vi "MBDoE3ParamAmb.vi"() -> ()   [LabVIEW 2015]
uses:
  <vilib>/Platform/TimedLoop/XDataNode/timing_clust.ctl
  <vilib>/Platform/TimedLoop/XDataNode/nitl_modes.ctl
  <vilib>/Platform/TimedLoop/XDataNode/wakeup.ctl
  <vilib>/DAQmx/read.llb/DAQmx Read (Analog DBL 1Chan 1Samp).vi
  <vilib>/DAQmx/read.llb/DAQmx Read (Analog 1D DBL NChan 1Samp).vi
  <vilib>/DAQmx/create/channels.llb/DAQmx Create Channel (AI-Voltage-Basic).vi
  <vilib>/Enthought/Python Integration Toolkit/api/Unpack Double.vi
  <vilib>/DAQmx/miscellaneous.llb/DAQmx Fill In Error Info.vi
  <vilib>/Platform/TimedLoop/XDataNode/XDataNode.xnode
  Program Files/neMESYS_SDK/neMESYS LabVIEW Kit/neMESYS LabVIEW Integration Kit.lvlib
  <vilib>/Platform/TimedLoop/XDataNode/XDNodeRunTimeDep.lvlib
  Conor/Temp CN7500/Omega CN7500/Omega CN7500.lvlib
  <vilib>/Enthought/Python Integration Toolkit/Python Integration Toolkit.lvlib
panel:
  in  "MBDoE Criteria A/D/E":string
  out "Record filename, RecordAmbInitisileFactorial1MD":string
  out "HPLC file name, MBDoE2peakin1":string
  out "Exp 9":bool
  out "Temp 9":dbl
  out "Flow 9":dbl
  out "Conc 9":dbl
  out "t1 - 8":dbl
  out "X2 ref A 8":dbl
  out "X2 B 8":dbl
  out "X ref B 8":dbl
  out "C BAcid 8":dbl
  out "C EB 8":dbl
  out "Exp 8":bool
  out "Temp 8":dbl
  out "Flow 8":dbl
  out "Conc 8":dbl
  out "t1 - 7":dbl
  out "X2 ref A 7":dbl
  out "X2 B 7":dbl
  out "X ref B 7":dbl
  out "C BAcid 7":dbl
  out "C EB 7":dbl
  out "Exp 7":bool
  out "Temp 7":dbl
  out "Flow 7":dbl
  out "Conc 7":dbl
  out "t1 - 6":dbl
  out "X2 ref A 6":dbl
  out "X2 B 6":dbl
  out "X ref B 6":dbl
  out "C BAcid 6":dbl
  out "C EB 6":dbl
  out "Exp 6":bool
  out "Temp 6":dbl
  out "Flow 6":dbl
  out "Conc 6":dbl
  out "t1 - 5":dbl
  out "X2 ref A 5":dbl
  out "X2 B 5":dbl
  out "X ref B 5":dbl
  out "C BAcid 5":dbl
  out "C EB 5":dbl
  out "Exp 5":bool
  out "Temp 5":dbl
  out "Flow 5":dbl
  out "Conc 5":dbl
  out "t1 - 4":dbl
  out "X2 ref A 4":dbl
  out "X2 B 4":dbl
  out "X ref B 4":dbl
  out "C BAcid 4":dbl
  out "C EB 4":dbl
  out "Exp 4":bool
  out "Temp 4":dbl
  out "Flow 4":dbl
  out "Conc 4":dbl
  out "t1 - 3":dbl
  out "X2 ref A 3":dbl
  out "X2 B 3":dbl
  out "X ref B 3":dbl
  out "C BAcid 3":dbl
  out "C EB 3":dbl
  out "Exp 3":bool
  out "Temp 3":dbl
  out "Flow 3":dbl
  out "Conc 3":dbl
  out "t1 2":dbl
  out "X2 ref A 2":dbl
  out "X2 B 2":dbl
  out "X ref B 2":dbl
  out "C BAcid 2":dbl
  out "C EB 2":dbl
  in  "Cat Mass (0.096 g)":dbl
  in  "Cat Diameter (825 um)":dbl
  out "t1 - 1":dbl
  out "X2 ref A 1":dbl
  out "X2 B 1":dbl
  out "X ref B 1":dbl
  out "Exp 1":bool
  out "C EB 1":dbl
  out "C BAcid 1":dbl
  out "Liquid Inlet Pressure (bar g)":dbl
  in  "Liquid P sensor Terminal Configuration":i32(ring)=-1 items=["default"=-1, "RSE"=10083, "NRSE"=10078, "Differential"=10106, "Pseudodifferential"=12529]
  in  "Liquid P sensor Physical Channel":tag="Dev1/ai0"
  out "Exp 2":bool
  out "Exp 0":bool
  out "Conc 1":dbl
  out "Flow 1":dbl
  out "Temp 1":dbl
  out "Conc 2":dbl
  out "Flow 2":dbl
  out "Temp 2":dbl
  out "t1":dbl
  out "t2":dbl
  out "t3":dbl
  out "tref":dbl
  out "Desired Conc Not Possible":bool
  in  "Safety or Emergency Syringe Control":bool
  out "Feed Concentration (M)":dbl
  out "Total Flowrate (uL/min)":dbl
  out "Gas Back Pressure (barg)":dbl
  in  "Shut down in empty?\nLeft off, right on":bool
  in  "Clear":bool
  out "Safety Shut Down Pressure (barg)":dbl
  out "Calculated Pressure":dbl[](graph)
  out "Safety Shut Down Temp":dbl
  out "Actual Temp (oC)":dbl
  out "Temperature":dynamicdata(graph)
  out "Temp Set Point (oC)":dbl
  in  "Temp 0":dbl
  in  "Update Temperature Set Point":bool
  in  "Automated Experiments or Direct Control":bool
  in  "Set Point (oC)":dbl
  out "loop ind":dbl
  in  "Stop everything":bool
  in  "Skip Exp":bool
  in  "Minutes between Exp":dbl min=0.0 step=0.05
  in  "Refill 4":bool
  in  "Refill 3":bool
  in  "Refill 2":bool
  in  "Refill 1":bool
  in  "Empty 4":bool
  in  "Empty 3":bool
  in  "Empty 2":bool
  in  "Empty 1":bool
  in  "Calibrate 4":bool
  in  "Calibrate 3":bool
  in  "Calibrate 2":bool
  in  "Calibrate 1":bool
  in  "Stop Dose 4":bool
  in  "Stop Dose 3":bool
  in  "Stop Dose 2":bool
  in  "Stop Dose 1":bool
  in  "Flow 0":dbl
  in  "Conc 0":dbl
  in  "Generate Flow":bool
  in  "Set Flowrate 1":dbl
  in  "Set Flowrate 2":dbl
  in  "Set Flowrate 3":dbl
  in  "Set Flowrate 4":dbl
  in  "High Conc":dbl min=0.0 max=2.0
  in  "Low Conc":dbl min=0.0 max=2.0
  out "Syringe Level 4":dbl(slide) scale=0.0..5500.0
  out "Syringe Level 3":dbl(slide) scale=0.0..5500.0
  out "Syringe Level 2":dbl(slide) scale=0.0..5500.0
  out "Syringe Level 1":dbl(slide) scale=0.0..5500.0
  out "Flowrate 4 High":dbl
  out "Flowrate 3 High":dbl
  out "Flowrate 2 Low":dbl
  out "Flowrate 1 Low":dbl
  # "Pre Planned Experiments"
  # "Conducted Experiments Set Points"
  # "Safety (start and end)"
  # "Current Conditions"
  # "(uL/min)"
  # "Coerced to nearest possible"
  # "Experimental Info"
  # "This code only does Automated \nDirect control just sets all variables to 0"
  # "Direct Control"
  # "Unit of Gas Flow NmL/min"
  # "Emergency Syringe Control Below"
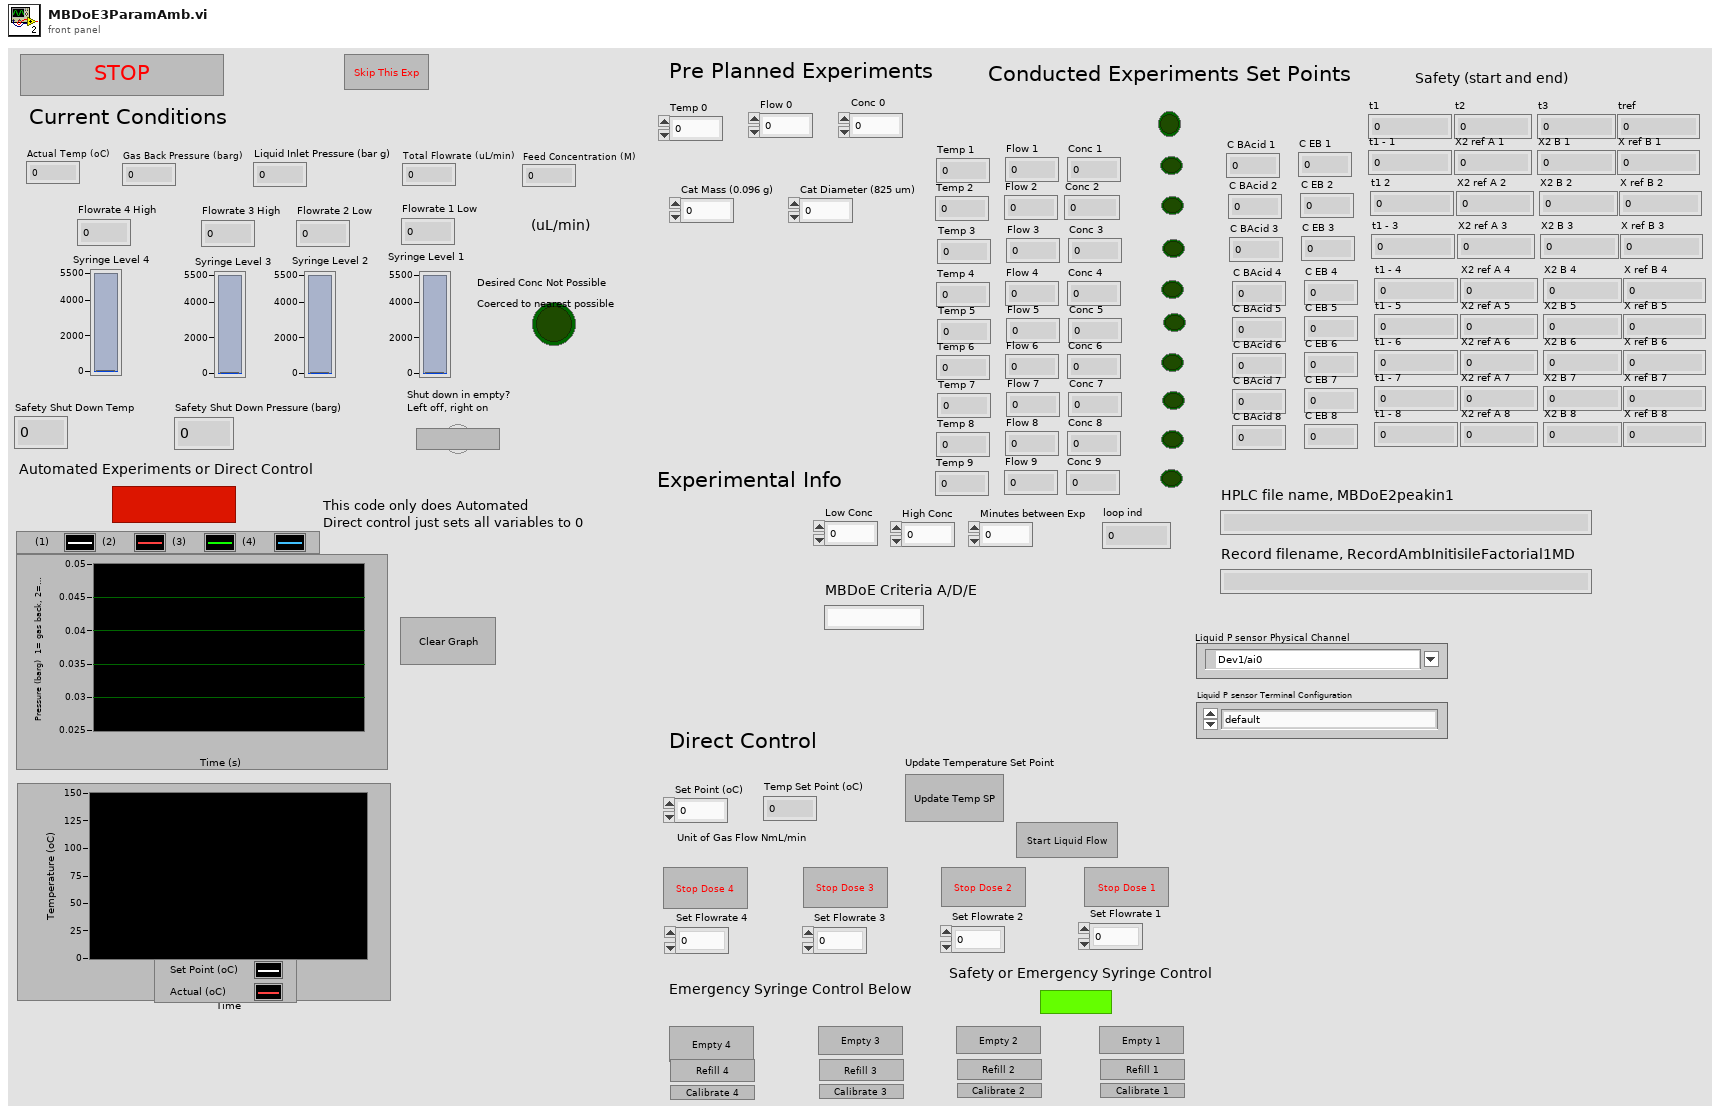
[diagram p1: front panel]
types:
  T1 = typedef "XDNodeRunTimeDep.lvlib/timing_clust.ctl" = cluster{"Expected End [f-1]":u64, "Actual End [f-1]":u64, "Finished Late? [f-1]":bool, "Expected End [i-1]":u64, "Actual End [i-1]":u64, "Finished Late? [i-1]":bool, "Expected Start [i]":u64, "Actual Start [i]":u64, "Expected Start [f]":u64, "Actual Start [f]":u64, "Source Name":string, "Structure Name":string, "Period":i64, "Deadline":i64, "Offset":i64, "Start":i64, "Priority":i32, "Timeout":i32, "Mode":T2, "Wakeup Reason":T3, "Error":errorcluster, "Source Type":string, "Secondary Source Type":string, "Global End Time":u64, "Global Start Time":u64, "Frame Duration":u64, "Iteration Duration":u64, "Assigned CPU":i32, "I/O Scan Engine Mode":u32}
  T2 = typedef "XDNodeRunTimeDep.lvlib/nitl_modes.ctl" = enum32{"No Change", "Process missed periods, maintain original phase", "Discard missed periods, maintain original phase", "Process missed periods, ignore original phase", "Discard missed periods, ignore original phase"}
  T3 = typedef "XDNodeRunTimeDep.lvlib/wakeup.ctl" = enum32{"Normal", "Aborted", "Asynchronous wakeup", "Timing source error", "Timed loop error", "Timeout"}
  T4 = typedef "Python Integration Toolkit.lvlib/Session ID.ctl" = u64
  T5 = typedef "Python Integration Toolkit.lvlib/Python Objects.ctl" = variant
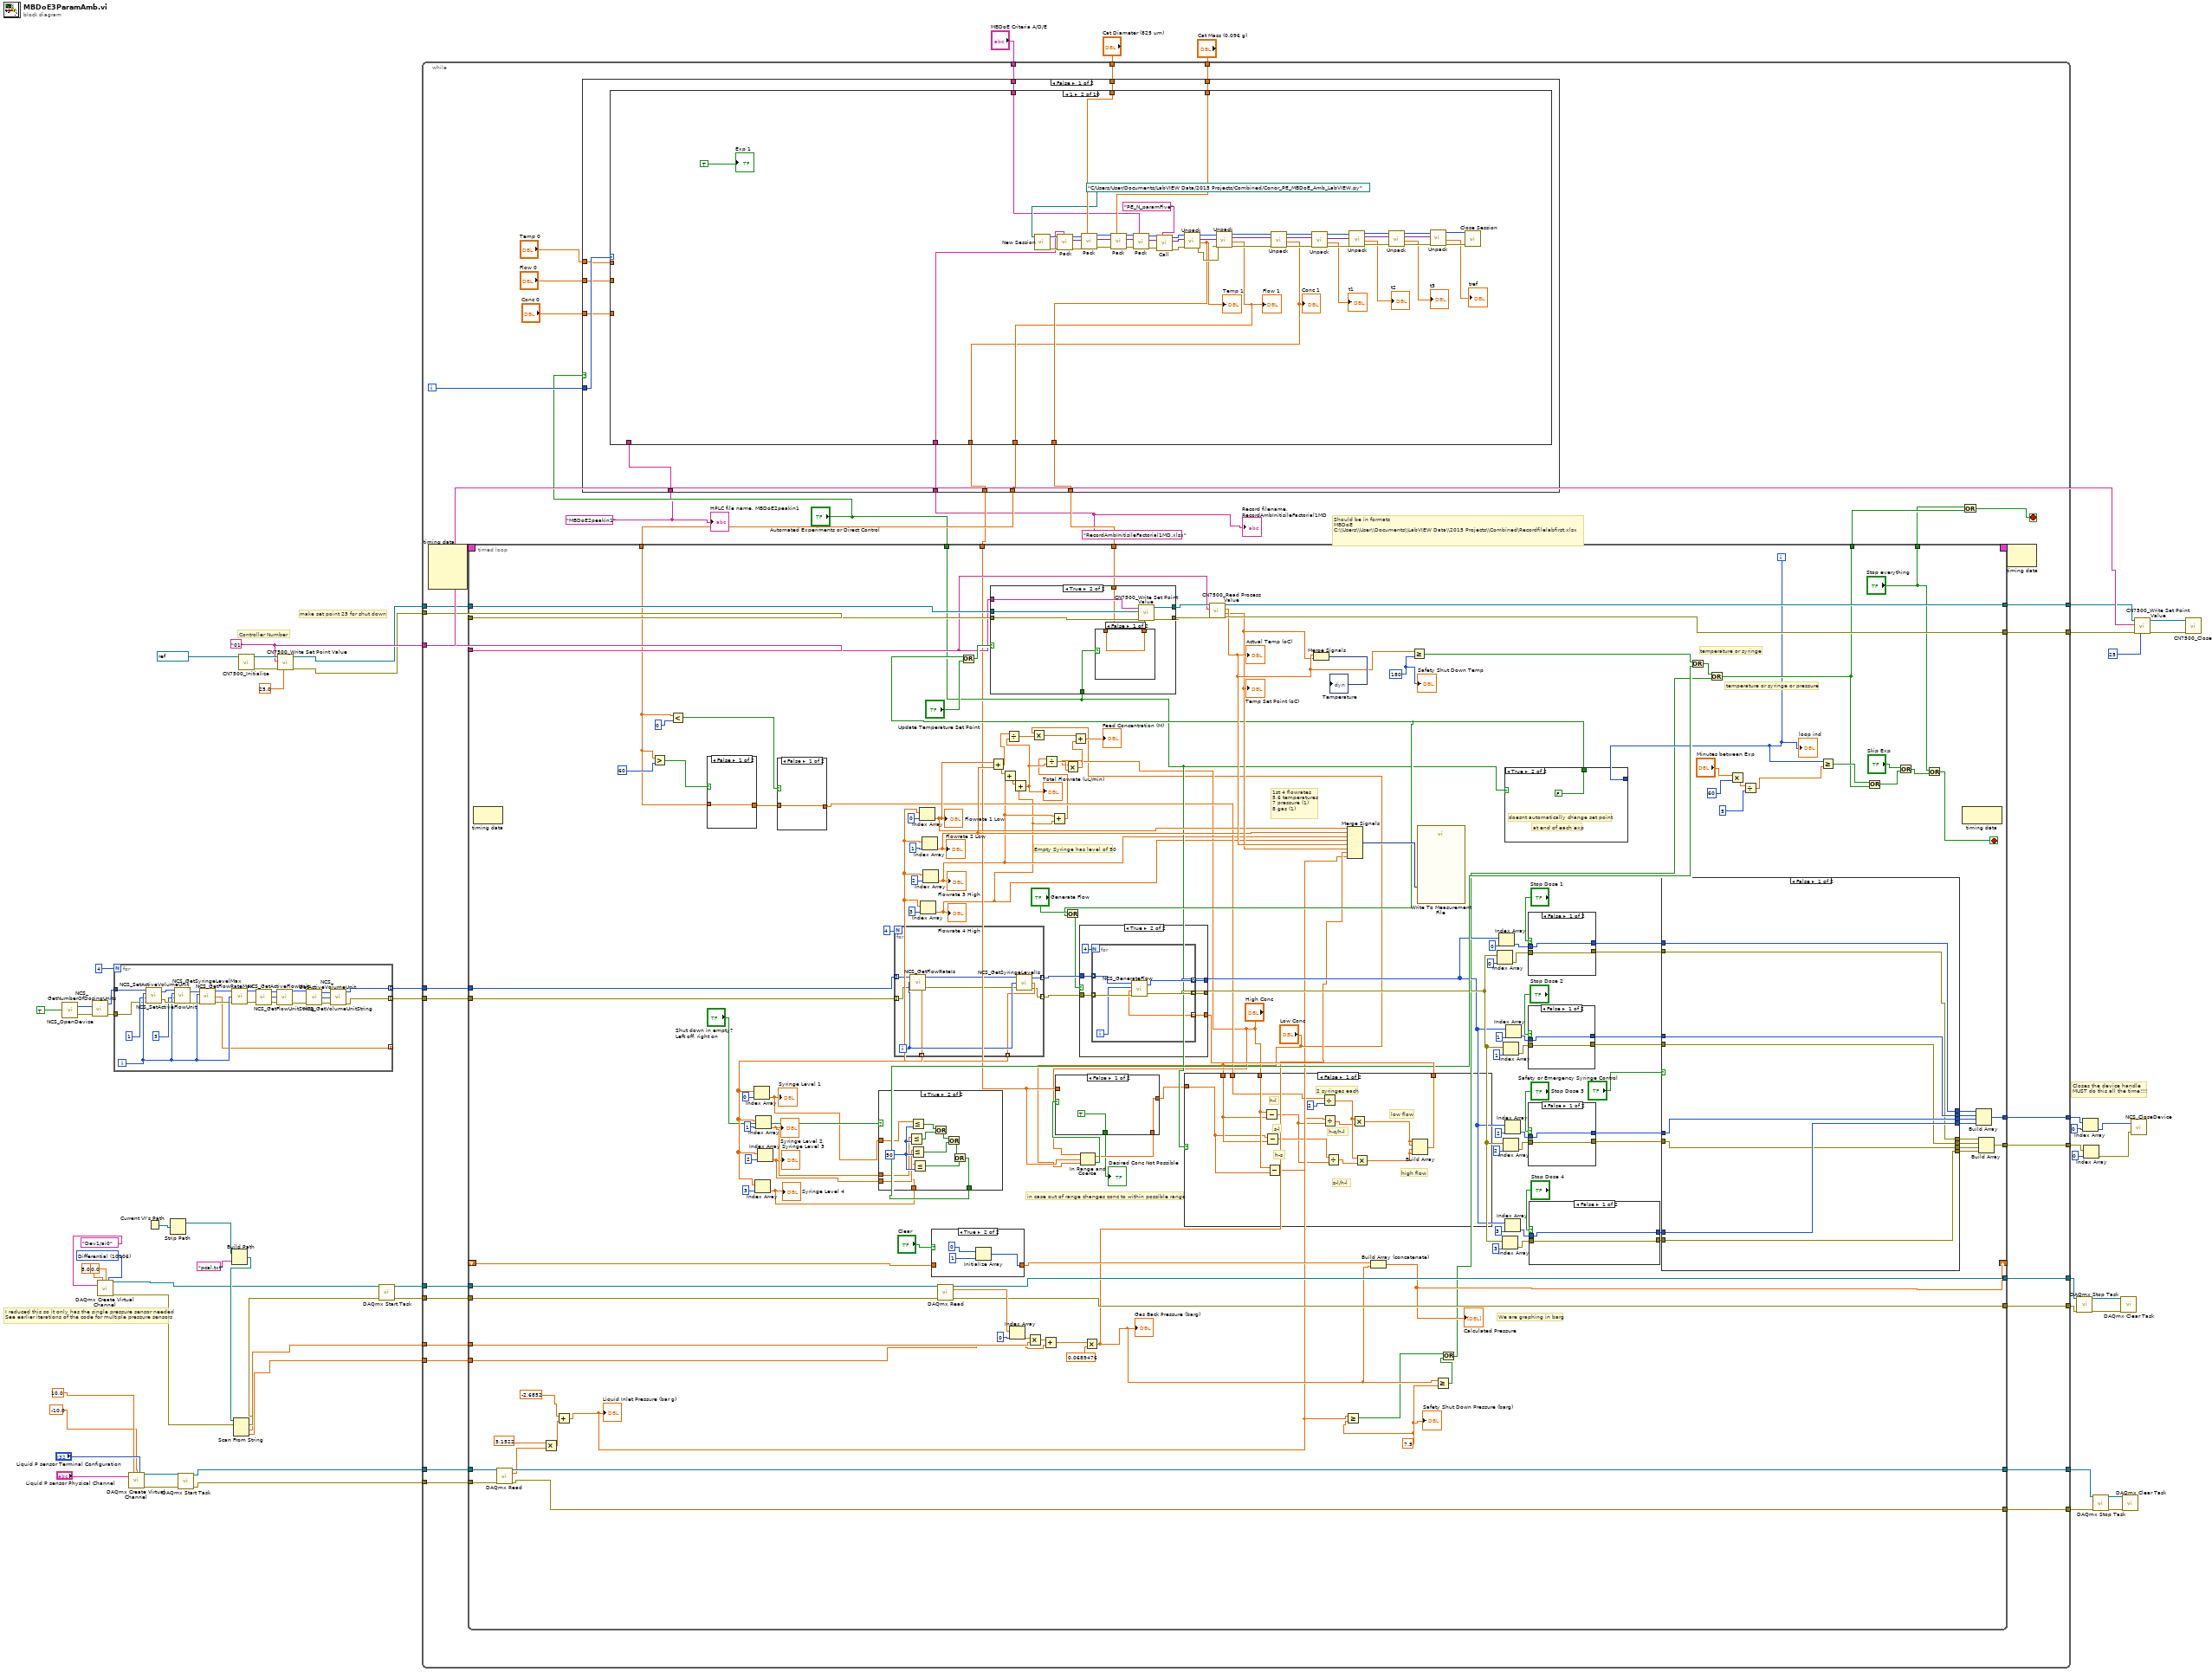
[diagram p0: block diagram]
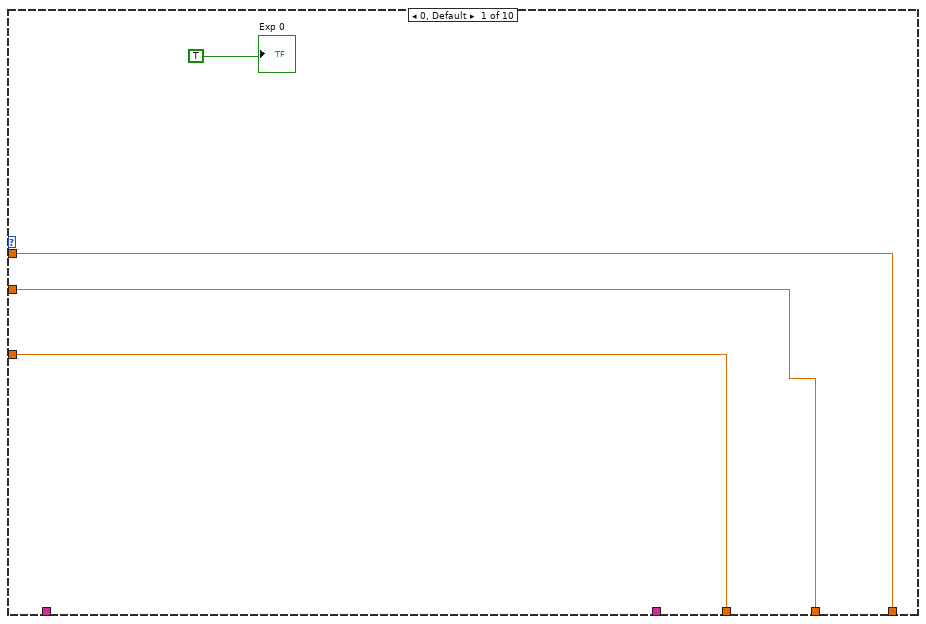
[diagram p2: hidden frame]
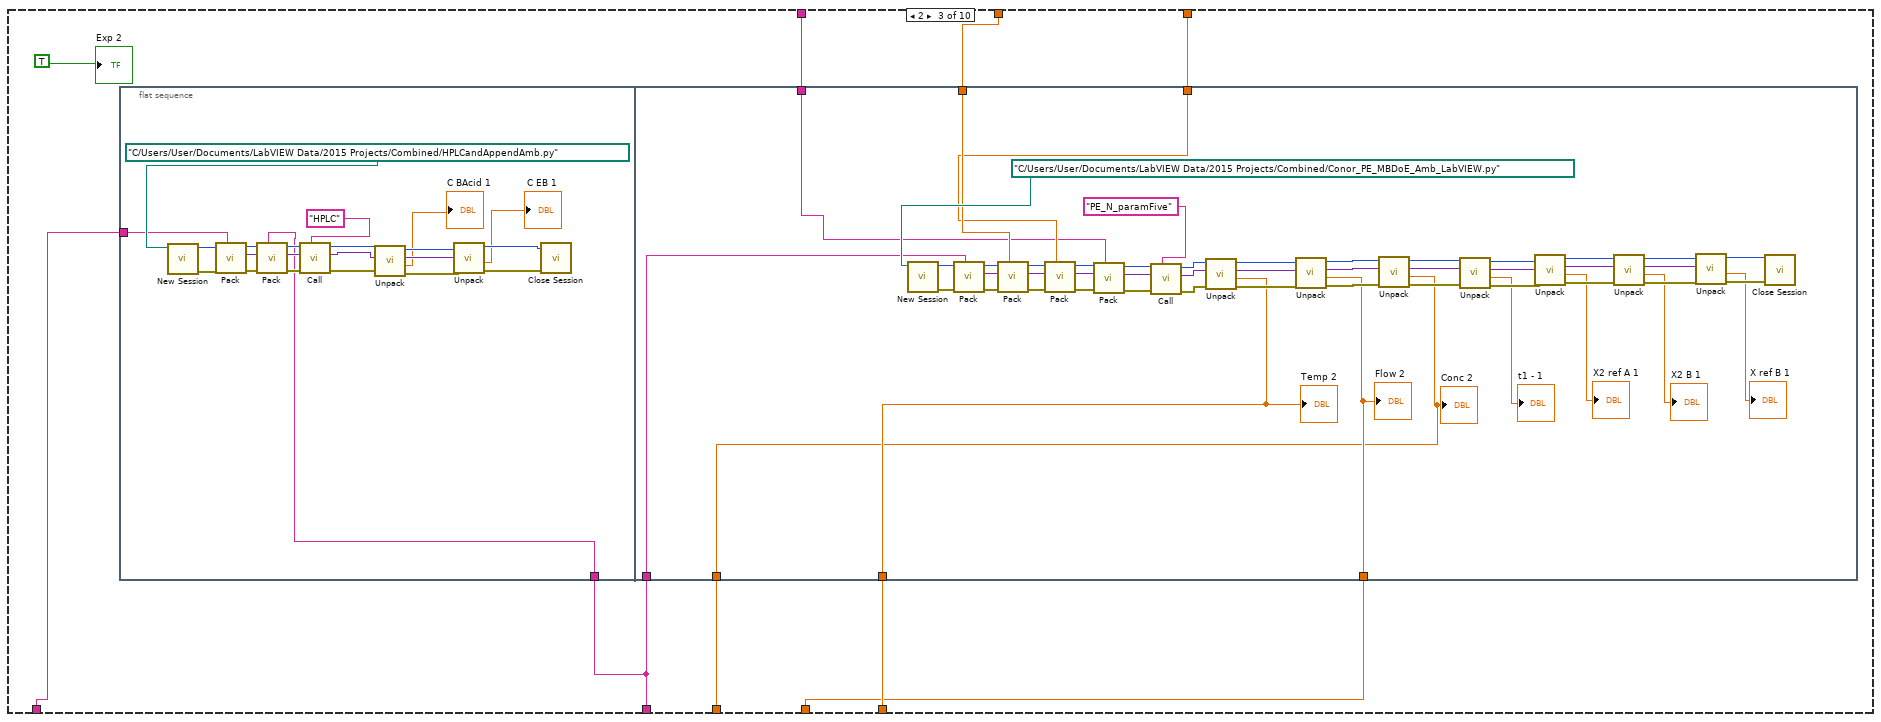
[diagram p3: hidden frame]
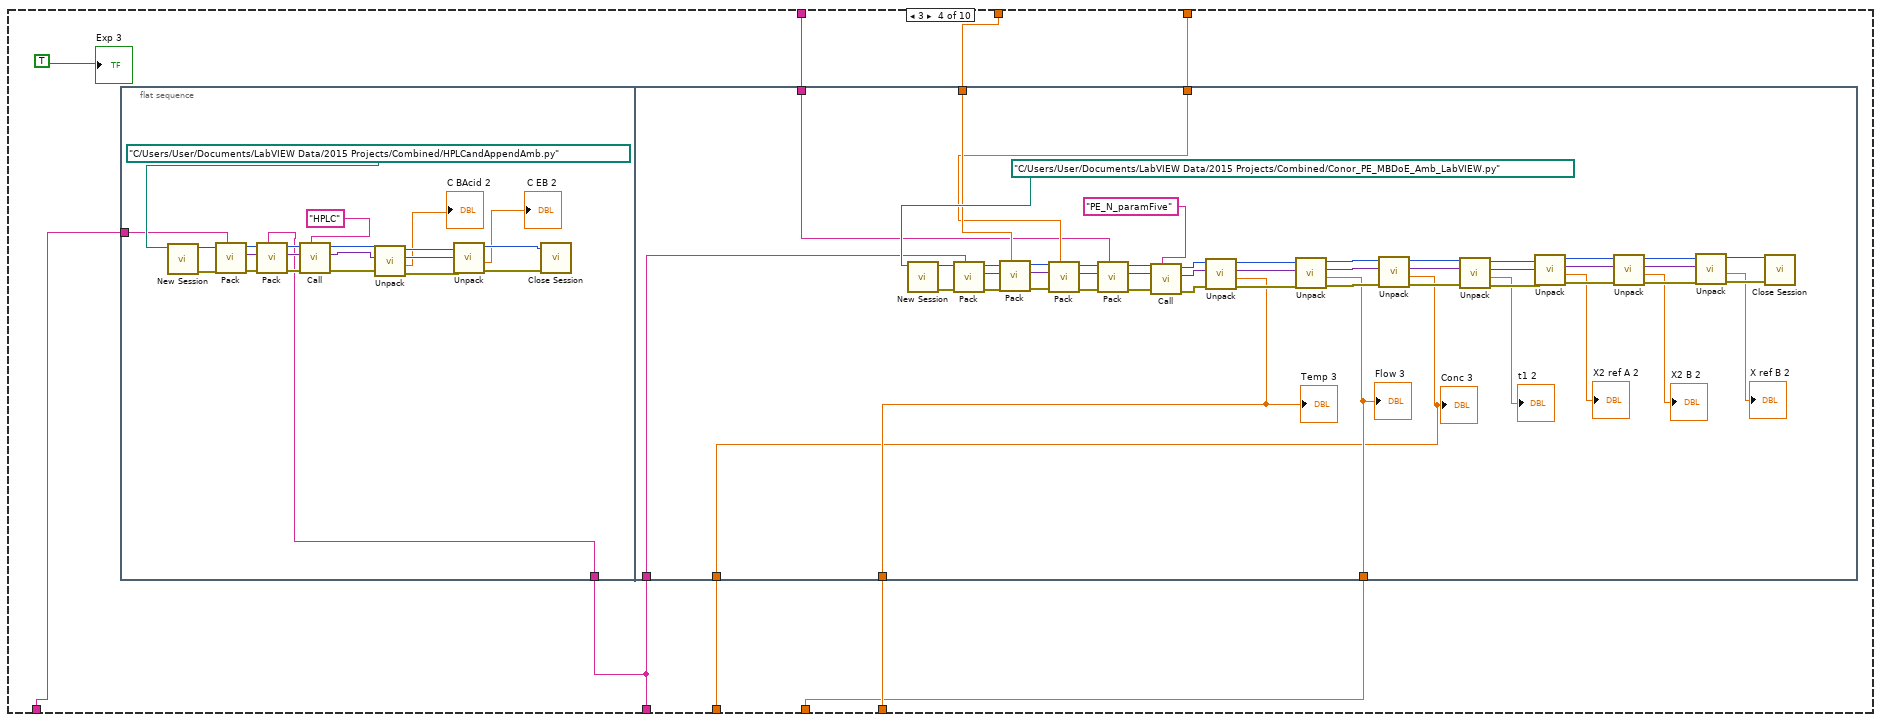
[diagram p4: hidden frame]
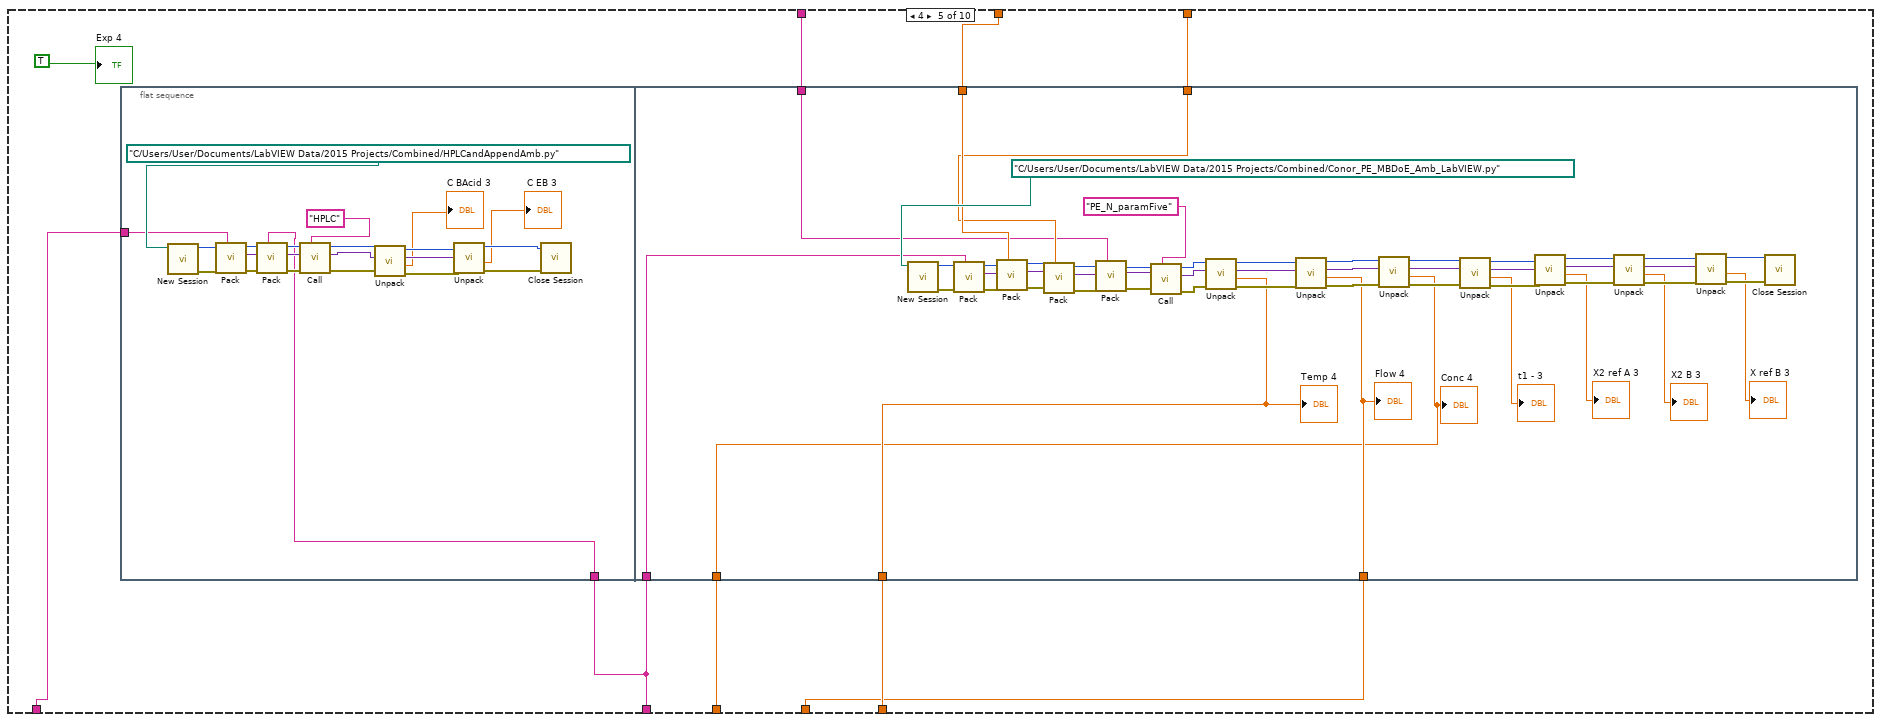
[diagram p5: hidden frame]
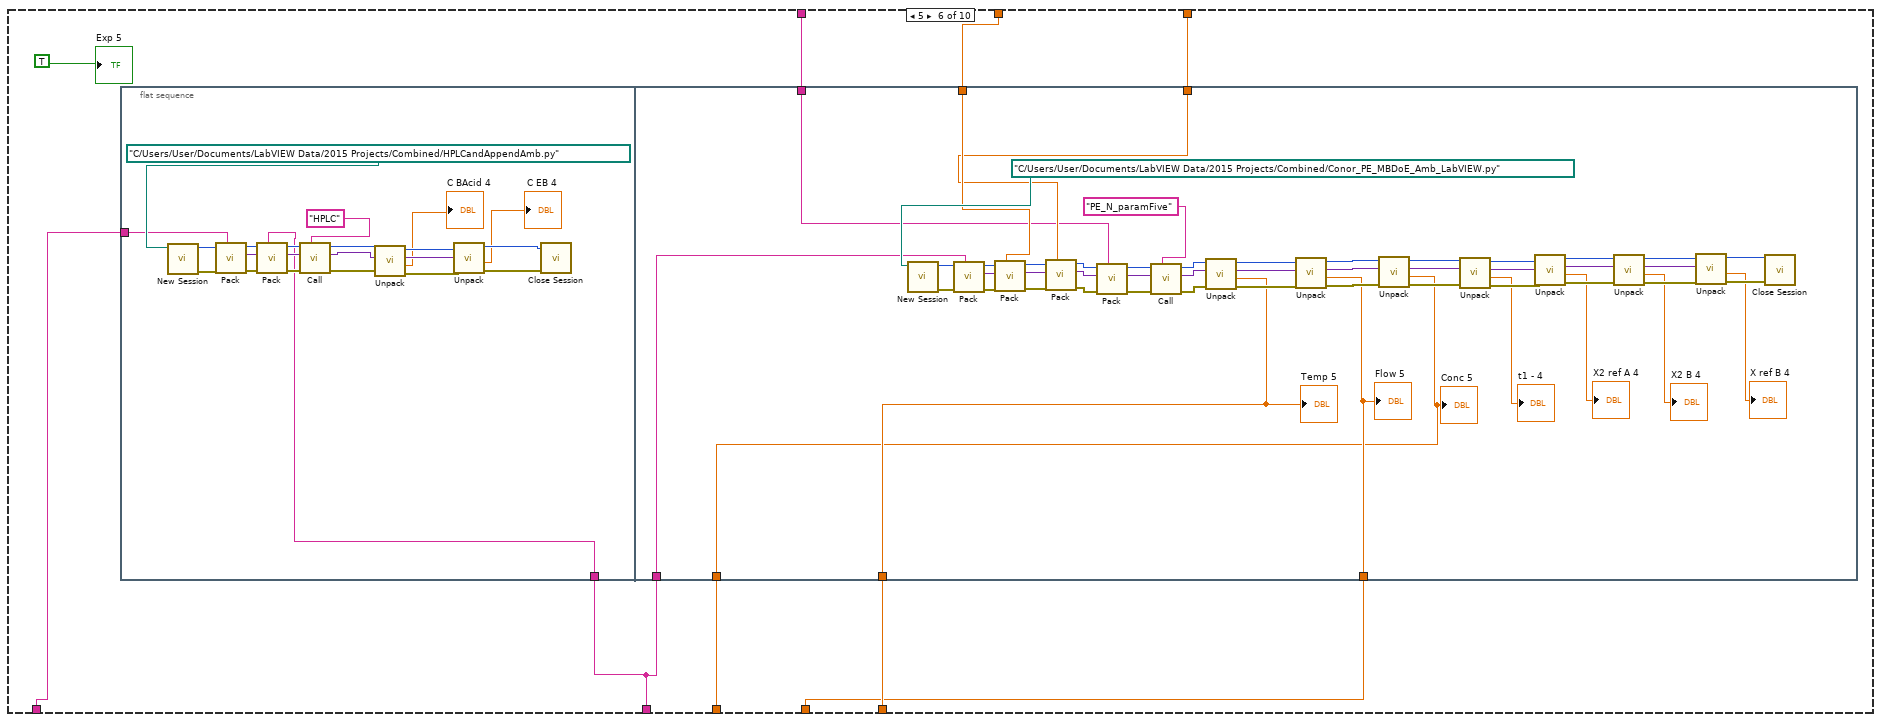
[diagram p6: hidden frame]
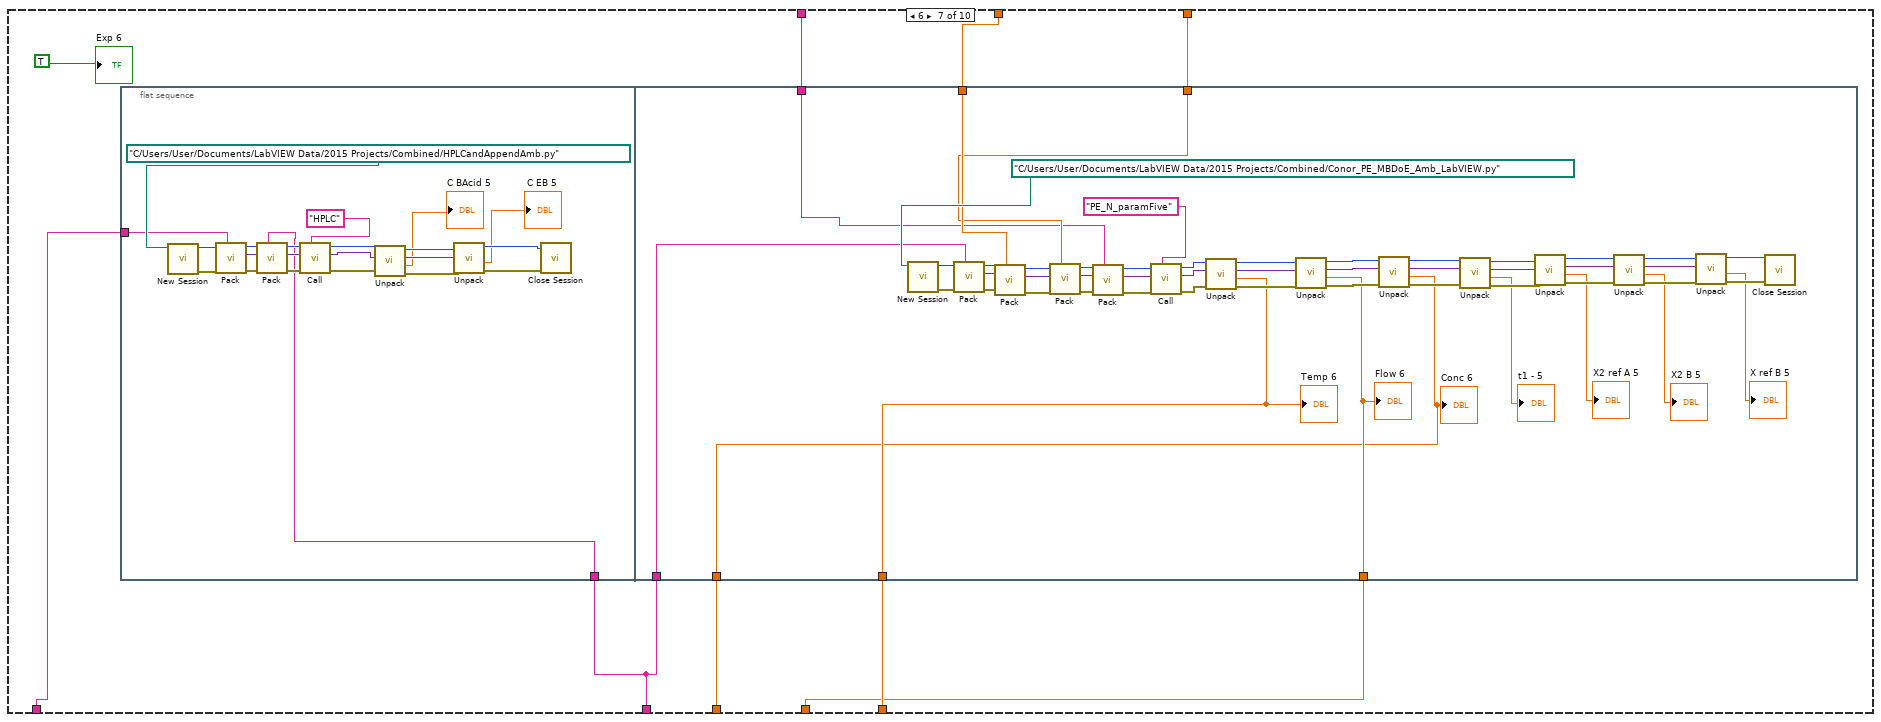
[diagram p7: hidden frame]
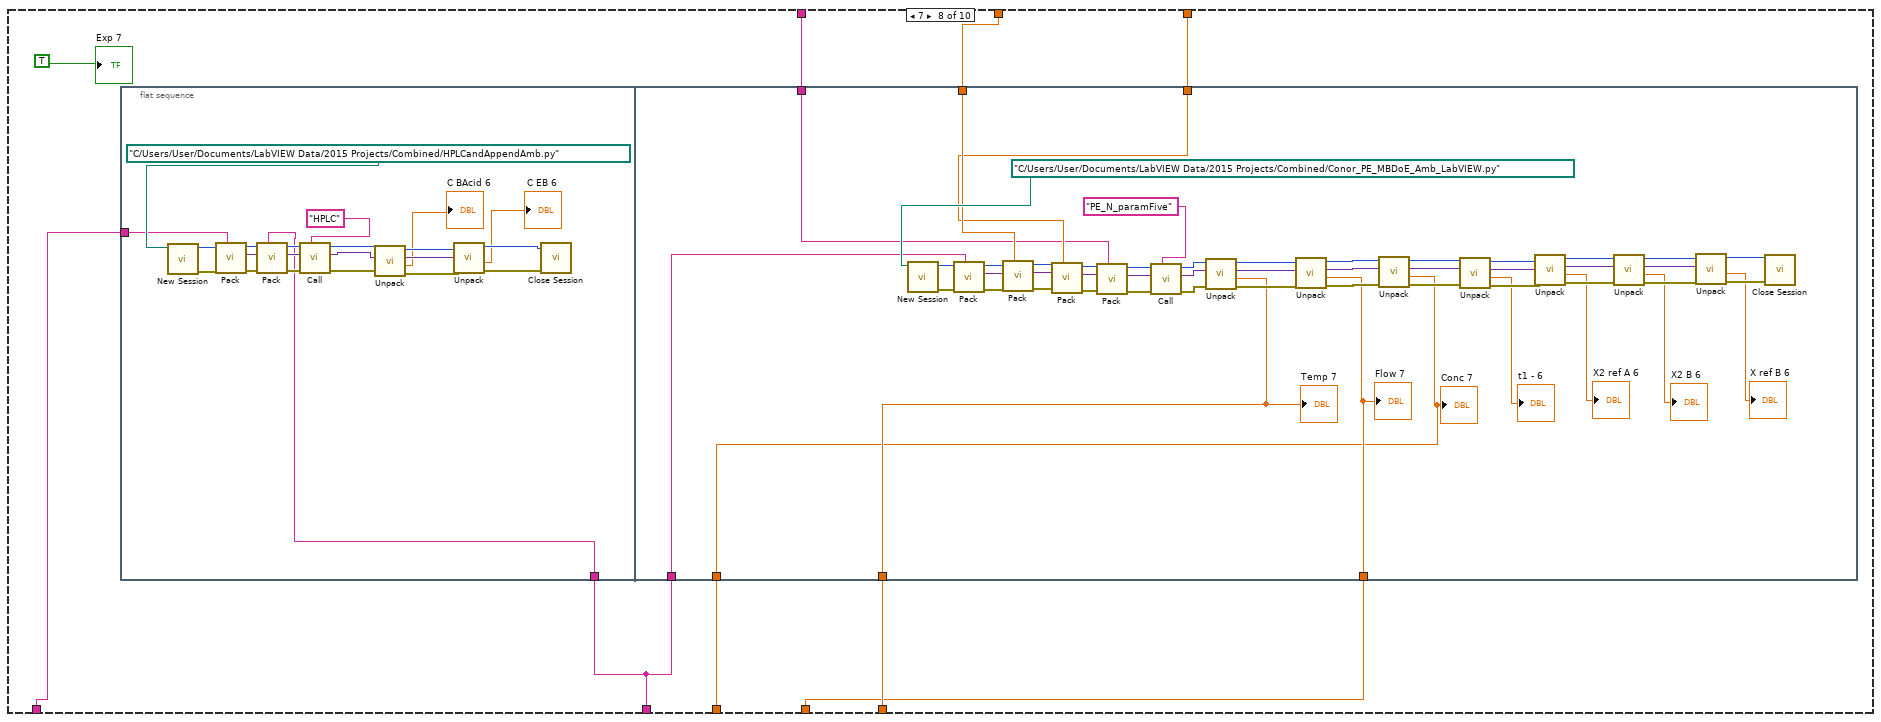
[diagram p8: hidden frame]
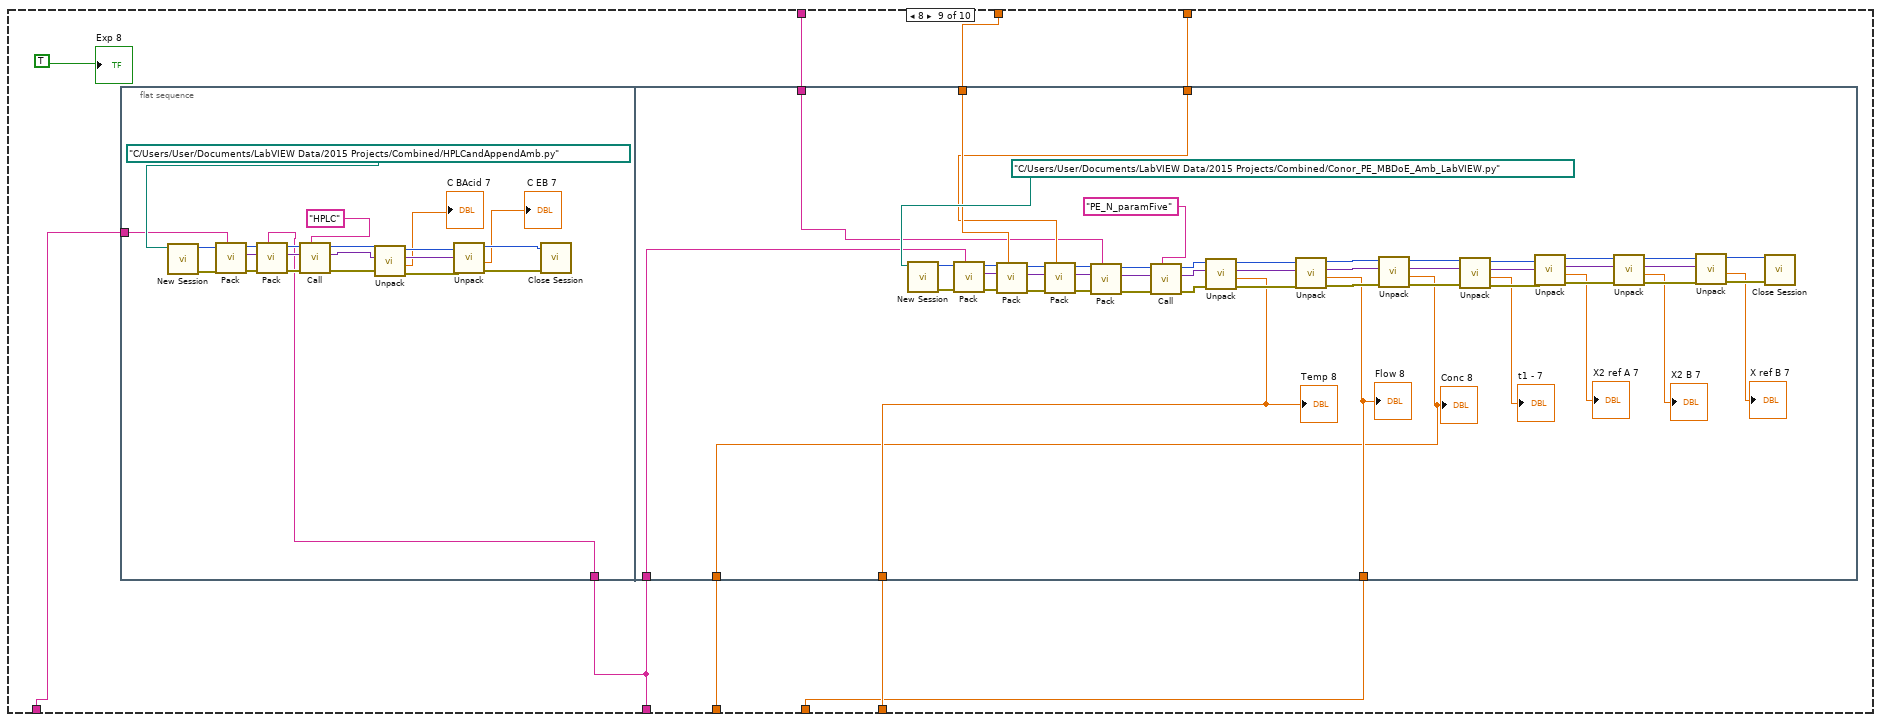
[diagram p9: hidden frame]
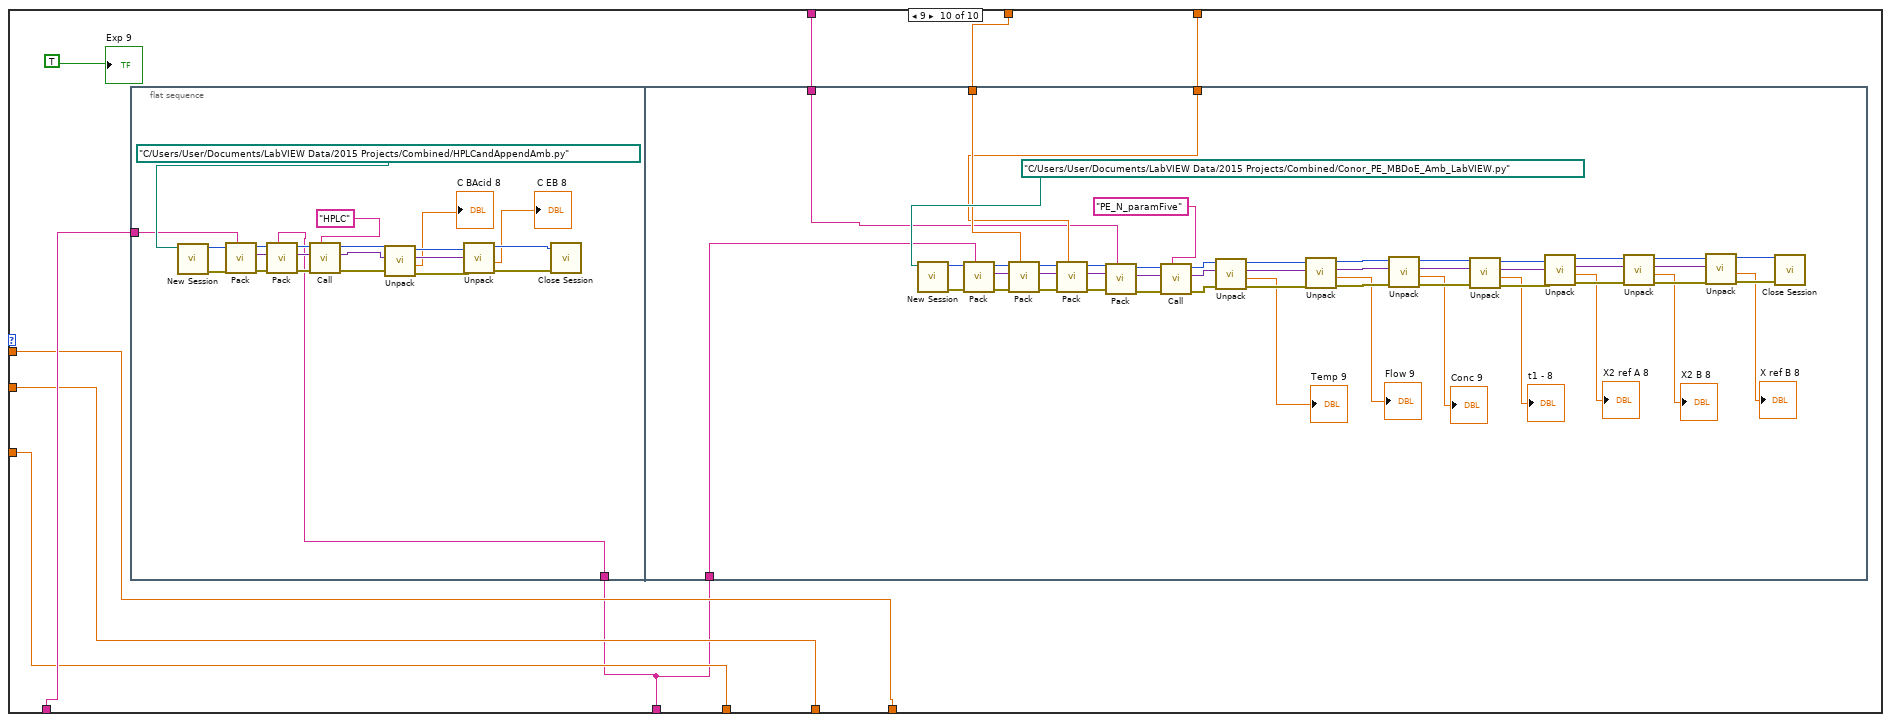
[diagram p10: hidden frame]
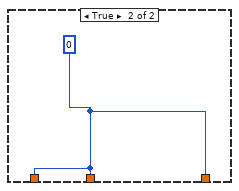
[diagram p11: hidden frame]
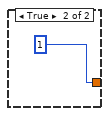
[diagram p12: hidden frame]
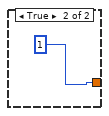
[diagram p13: hidden frame]
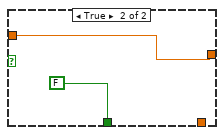
[diagram p14: hidden frame]
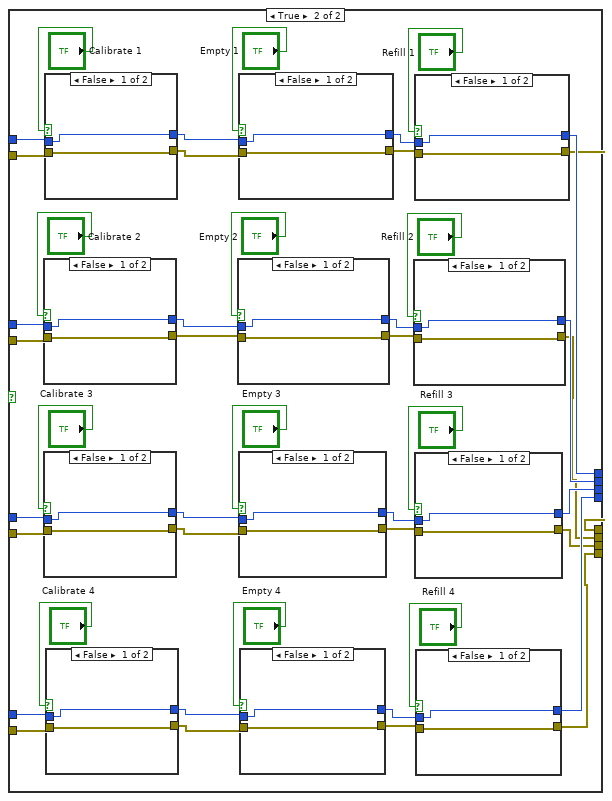
[diagram p15: hidden frame]
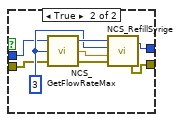
[diagram p16: hidden frame]
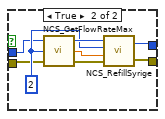
[diagram p17: hidden frame]
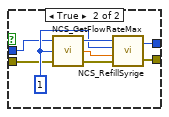
[diagram p18: hidden frame]
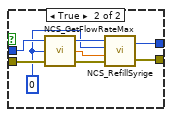
[diagram p19: hidden frame]
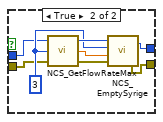
[diagram p20: hidden frame]
diagram:
  w32 = 10106 items=["default"=-1, "RSE"=10083, "NRSE"=10078, "Differential"=10106, "Pseudodifferential"=12529] ("input terminal configuration")
  w39 = "01" ("Controller Number")
  # "I reduced this so it only has the single pressure sensor needed\nSee earlier iterations of the code for multiple pressure sensors"
  # "make set point 25 for shut down"
  # "Controller Number"
  # "Closes the device handle \nMUST do this all the time!!!!"
  n1 = call "NCS_OpenDevice.vi"("show status window"=TRUE) -> ("device handle"=w58:u32, "error out"=w57:errorcluster)
  n2 = call "NCS_GetNumberOfDosingUnits.vi"("device handle in"=w58, "error in (no error)"=w57) -> ("device handle out"=w55:u32, "error out"=w56:errorcluster)  [unwired: 1 out]
  n3 = call-poly <vilib>:"DAQmx Create Virtual Channel.vi"("maximum value"=5.0, "minimum value"=0.0, "input terminal configuration"=w32, "physical channels"=tag "Dev1/ai0") -> ("task out"=w16:refnum<k21>, "error out"=w17:errorcluster)  [unwired: 10 in]
  n4 = for {
    N: 4 -> [_]
    tunnel: [w64] -> w54 mode=indexing
    tunnel: [w63] -> w53 mode=indexing
    tunnel: [w77] -> _ mode=indexing
    tunnel: w56 -> [w62]
    tunnel: w55 -> [w61]
    i -> [w80]
    n5 = call "NCS_SetActiveVolumeUnit.vi"("error in (no error)"=w62, "active volume unit"=1, "dosingunit"=w80, "device handle in"=w61) -> ("error out"=w83:errorcluster, "device handle out"=w84:u32)
    n6 = call "NCS_SetActiveFlowUnit.vi"("error in (no error)"=w83, "active flow unit"=3, "dosingunit"=w80, "device handle in"=w84) -> ("error out"=w81:errorcluster, "device handle out"=w82:u32)
    n7 = call "NCS_GetSyringeLevelMax.vi"("error in (no error)"=w81, "dosingunit"=w80, "device handle in"=w82) -> ("error out"=w78:errorcluster, "syringe level max"=w77:dbl, "device handle out"=w79:u32)  [unwired: 1 out]
    n8 = call "NCS_GetFlowRateMax.vi"("error in (no error)"=w78, "dosingunit"=w80, "device handle in"=w79) -> ("error out"=w65:errorcluster, "device handle out"=w66:u32)  [unwired: 1 out]
    n9 = call "NCS_GetActiveFlowUnit.vi"("error in (no error)"=w65, "device handle in"=w66) -> ("error out"=w73:errorcluster, "active flow unit"=w72:u8, "device handle out"=w74:u32)  [unwired: 1 in]
    n10 = call "NCS_GetFlowUnitString.vi"("device handle in"=w74, "flow unit id"=w72, "error in (no error)"=w73) -> ("device handle out"=w69:u32, "error out"=w68:errorcluster)  [unwired: 2 out]
    n11 = call "NCS_GetActiveVolumeUnit.vi"("error in (no error)"=w68, "device handle in"=w69) -> ("error out"=w70:errorcluster, "active volume unit"=w71:u8, "device handle out"=w67:u32)  [unwired: 1 in]
    n12 = call "NCS_GetVolumeUnitString.vi"("device handle in"=w67, "volume unit id"=w71, "error in (no error)"=w70) -> ("device handle out"=w64:u32, "error out"=w63:errorcluster)  [unwired: 2 out]
  }
  n13 = call-poly <vilib>:"DAQmx Create Virtual Channel.vi"("maximum value"=10.0, "minimum value"=-10.0 ("maximum value"), "input terminal configuration"="Liquid P sensor Terminal Configuration", "physical channels"="Liquid P sensor Physical Channel") -> ("task out"=w12:refnum<k21>, "error out"=w13:errorcluster)  [unwired: 10 in]
  n14 = Current VI's Path() -> (path=w30:path)
  n15 = Strip Path(path=w30) -> (stripped path=w28:path)  [unwired: 1 out]
  n16 = call <vilib>:"DAQmx Start Task.vi"("task/channels in"=w12, "error in"=w13) -> ("task out"=w11:refnum<k21>, "error out"=w10:errorcluster)  [unwired: 12 in]
  n17 = Build Path(base path=w28, name or relative path="pcal.txt") -> (appended path=w29:path)
  n18 = Scan From String(w29, w17) -> (w26:errorcluster, output 1=w23:dbl, output 2=w22:dbl)  [unwired: 3 in, 1 out]
  n19 = call "CN7500_Initialize.vi"("VISA resource name"=refnum<visa-resource-name> "COM8") -> ("error out"=w45:errorcluster, "VISA resource name out"=w46:refnum<visa-resource-name>)  [unwired: 9 in]
  n20 = call "CN7500_Write Set Point Value.vi"("Target Set Point Value"=25.0, "error in (no error)"=w45, "Controller Number"=w39, "VISA In"=w46) -> ("error out"=w37:errorcluster, "VISA Out"=w38:refnum<visa-resource-name>)  [unwired: 6 in]
  n21 = call <vilib>:"DAQmx Start Task.vi"("task/channels in"=w16, "error in"=w26) -> ("task out"=w25:refnum<k21>, "error out"=w24:errorcluster)  [unwired: 12 in]
  n22 = while {
    tunnel: w54 -> [w121]
    tunnel: w53 -> [w120]
    tunnel: [w119] -> w48
    tunnel: [w118] -> w47
    tunnel: w39 -> [w115]
    tunnel: w38 -> [w114]
    tunnel: w37 -> [w113]
    tunnel: [w112] -> w36
    tunnel: [w111] -> w35
    tunnel: w25 -> [w109]
    tunnel: w24 -> [w108]
    tunnel: w23 -> [w107]
    tunnel: w22 -> [w106]
    tunnel: [w105] -> w19
    tunnel: [w104] -> w18
    tunnel: w11 -> [w93]
    tunnel: w10 -> [w92]
    tunnel: [w91] -> w8
    tunnel: [w90] -> w6
    tunnel: "Cat Diameter (825 um)" -> [w89]
    tunnel: "Cat Mass (0.096 g)" -> [w88]
    tunnel: "MBDoE Criteria A/D/E" -> [w85]
    i -> [w98]
    stop <- w103 stop-if-true
    w86 = "RecordAmbInitisileFactorial1MD.xlsx" ("Result file name must end with .xlsx")
    w87 = "MBDoE2peakin1" ("HPLC file Name, dont need extension")
    # "Should be in formats \nMBDoE\nC:\\\\Users\\\\User\\\\Documents\\\\LabVIEW Data\\\\2015 Projects\\\\Combined\\Recordfilelabfirst.xlsx"
    n23 = node-c288() -> (w117:T1)  [unwired: 4 in]
    n24 = case shown="False" "Automated Experiments or Direct Control" {
      tunnel: [w130 w837] -> w101
      tunnel: [w128 w837] -> w100
      tunnel: [w132 w837] -> w99
      tunnel: w98 -> [w133 _]
      tunnel: "Conc 0" -> [w131 _]
      tunnel: "Flow 0" -> [w127 _]
      tunnel: "Temp 0" -> [w129 _]
      tunnel: w87 -> [w125 _]
      tunnel: w86 -> [w126 _]
      tunnel: w89 -> [w124 _]
      tunnel: w88 -> [w123 _]
      tunnel: w85 -> [w122 _]
      frame False {
        n25 = case shown="1" w133 {
          tunnel: [w135 w145 w193 w274 w355 w436 w517 w598 w679 w760] -> w132
          tunnel: w131 -> [w135 _ _ _ _ _ _ _ _ w760]
          tunnel: [w137 w147 w195 w276 w357 w438 w519 w600 w681 w762] -> w130
          tunnel: w129 -> [w137 _ _ _ _ _ _ _ _ w762]
          tunnel: [w136 w146 w194 w275 w356 w437 w518 w599 w680 w761] -> w128
          tunnel: w127 -> [w136 _ _ _ _ _ _ _ _ w761]
          tunnel: w126 -> [_ w152 w192 w273 w354 w435 w516 w597 w678 w759]
          tunnel: w125 -> [_ _ w196 w277 w358 w439 w520 w601 w682 w763]
          tunnel: w124 -> [_ w155 w191 w272 w353 w434 w515 w596 w677 w758]
          tunnel: w123 -> [_ w154 w190 w271 w352 w433 w514 w595 w676 w757]
          tunnel: w122 -> [_ w138 w189 w270 w351 w432 w513 w594 w675 w756]
          frame 0, Default {
            "Exp 0" <- TRUE
          }
          frame 1 {
            n26 = call <vilib>:"New Session.vi"("Path to Python Module (.py File)"=path "C:/Users/User/Documents/LabVIEW Data/2015 Projects/Combined/Conor_PE_MBDoE_Amb_LabVIEW.py") -> ("error out"=w180:errorcluster, "Session ID out"=w179:T4)  [unwired: 9 in]
            n27 = call <vilib>:"Pack.vi"("Argument"=w152, "error in (no error)"=w180, "Session ID"=w179) -> ("error out"=w173:errorcluster, "Python Object References Out"=w174:T5, "Session ID out"=w175:T4)  [unwired: 6 in]
            n28 = call <vilib>:"Pack.vi"("Argument"=w155, "error in (no error)"=w173, "Python Object References In"=w174, "Session ID"=w175) -> ("error out"=w158:errorcluster, "Python Object References Out"=w160:T5, "Session ID out"=w159:T4)  [unwired: 5 in]
            n29 = call <vilib>:"Pack.vi"("Argument"=w154, "error in (no error)"=w158, "Python Object References In"=w160, "Session ID"=w159) -> ("error out"=w140:errorcluster, "Python Object References Out"=w142:T5, "Session ID out"=w144:T4)  [unwired: 5 in]
            n30 = call <vilib>:"Pack.vi"("Argument"=w138, "error in (no error)"=w140, "Python Object References In"=w142, "Session ID"=w144) -> ("error out"=w139:errorcluster, "Python Object References Out"=w141:T5, "Session ID out"=w143:T4)  [unwired: 5 in]
            n31 = call <vilib>:"Call.vi"("Function or Method Name"="PE_N_paramFive", "error in (no error)"=w139, "Python Object References In"=w141, "Session ID"=w143) -> ("error out"=w166:errorcluster, "Python Object References Out"=w169:T5, "Session ID out"=w172:T4)  [unwired: 5 in]
            n32 = call-poly <vilib>:"Unpack.vi"("error in (no error)"=w166, "Python Object References In"=w169, "Session ID"=w172) -> ("error out"=w165:errorcluster, "Value"=w147:dbl, "Python Object References Out"=w168:T5, "Session ID out"=w171:T4)  [unwired: 5 in]
            "Temp 1" <- w147
            n33 = call-poly <vilib>:"Unpack.vi"("error in (no error)"=w165, "Python Object References In"=w168, "Session ID"=w171) -> ("error out"=w164:errorcluster, "Value"=w146:dbl, "Python Object References Out"=w167:T5, "Session ID out"=w170:T4)  [unwired: 5 in]
            "Flow 1" <- w146
            n34 = call-poly <vilib>:"Unpack.vi"("error in (no error)"=w164, "Python Object References In"=w167, "Session ID"=w170) -> ("error out"=w161:errorcluster, "Value"=w145:dbl, "Python Object References Out"=w162:T5, "Session ID out"=w163:T4)  [unwired: 5 in]
            "Conc 1" <- w145
            n35 = call-poly <vilib>:"Unpack.vi"("error in (no error)"=w161, "Python Object References In"=w162, "Session ID"=w163) -> ("error out"=w185:errorcluster, "Value"=→"t1":dbl, "Python Object References Out"=w183:T5, "Session ID out"=w181:T4)  [unwired: 5 in]
            n36 = call-poly <vilib>:"Unpack.vi"("error in (no error)"=w185, "Python Object References In"=w183, "Session ID"=w181) -> ("error out"=w186:errorcluster, "Value"=→"t2":dbl, "Python Object References Out"=w184:T5, "Session ID out"=w182:T4)  [unwired: 5 in]
            n37 = call-poly <vilib>:"Unpack.vi"("error in (no error)"=w186, "Python Object References In"=w184, "Session ID"=w182) -> ("error out"=w187:errorcluster, "Value"=→"t3":dbl, "Python Object References Out"=w178:T5, "Session ID out"=w177:T4)  [unwired: 5 in]
            n38 = call-poly <vilib>:"Unpack.vi"("error in (no error)"=w187, "Python Object References In"=w178, "Session ID"=w177) -> ("error out"=w156:errorcluster, "Value"=→"tref":dbl, "Session ID out"=w157:T4)  [unwired: 5 in, 1 out]
            n39 = call <vilib>:"Close Session.vi"("error in (no error)"=w156, "Session ID"=w157) -> ()  [unwired: 9 in, 1 out]
            "Exp 1" <- TRUE
          }
          frame 2 {
            n40 = flat-sequence {
              tunnel: w196 -> [w207]
              tunnel: w192 -> [w200]
              tunnel: [w236] -> w195
              tunnel: [w235] -> w194
              tunnel: [w234] -> w193
              tunnel: w192 -> [w229]
              tunnel: w191 -> [w228]
              tunnel: w190 -> [w227]
              tunnel: w189 -> [w220]
              frame #0 {
                n41 = call <vilib>:"New Session.vi"("Path to Python Module (.py File)"=path "C:/Users/User/Documents/LabVIEW Data/2015 Projects/Combined/HPLCandAppendAmb.py") -> ("error out"=w216:errorcluster, "Session ID out"=w215:T4)  [unwired: 9 in]
                n42 = call <vilib>:"Pack.vi"("Argument"=w207, "error in (no error)"=w216, "Session ID"=w215) -> ("error out"=w202:errorcluster, "Python Object References Out"=w204:T5, "Session ID out"=w206:T4)  [unwired: 6 in]
                n43 = call <vilib>:"Pack.vi"("Argument"=w200, "error in (no error)"=w202, "Python Object References In"=w204, "Session ID"=w206) -> ("error out"=w201:errorcluster, "Python Object References Out"=w203:T5, "Session ID out"=w205:T4)  [unwired: 5 in]
                n44 = call <vilib>:"Call.vi"("Function or Method Name"="HPLC", "error in (no error)"=w201, "Python Object References In"=w203, "Session ID"=w205) -> ("error out"=w217:errorcluster, "Python Object References Out"=w208:T5, "Session ID out"=w209:T4)  [unwired: 5 in]
                n45 = call-poly <vilib>:"Unpack.vi"("error in (no error)"=w217, "Python Object References In"=w208, "Session ID"=w209) -> ("error out"=w218:errorcluster, "Value"=→"C BAcid 1":dbl, "Python Object References Out"=w213:T5, "Session ID out"=w212:T4)  [unwired: 5 in]
                n46 = call-poly <vilib>:"Unpack.vi"("error in (no error)"=w218, "Python Object References In"=w213, "Session ID"=w212) -> ("error out"=w219:errorcluster, "Value"=→"C EB 1":dbl, "Session ID out"=w214:T4)  [unwired: 5 in, 1 out]
                n47 = call <vilib>:"Close Session.vi"("error in (no error)"=w219, "Session ID"=w214) -> ()  [unwired: 9 in, 1 out]
              }
              frame #1 {
                n48 = call <vilib>:"New Session.vi"("Path to Python Module (.py File)"=path "C:/Users/User/Documents/LabVIEW Data/2015 Projects/Combined/Conor_PE_MBDoE_Amb_LabVIEW.py") -> ("error out"=w262:errorcluster, "Session ID out"=w261:T4)  [unwired: 9 in]
                n49 = call <vilib>:"Pack.vi"("Argument"=w229, "error in (no error)"=w262, "Session ID"=w261) -> ("error out"=w255:errorcluster, "Python Object References Out"=w256:T5, "Session ID out"=w257:T4)  [unwired: 6 in]
                n50 = call <vilib>:"Pack.vi"("Argument"=w228, "error in (no error)"=w255, "Python Object References In"=w256, "Session ID"=w257) -> ("error out"=w242:errorcluster, "Python Object References Out"=w244:T5, "Session ID out"=w243:T4)  [unwired: 5 in]
                n51 = call <vilib>:"Pack.vi"("Argument"=w227, "error in (no error)"=w242, "Python Object References In"=w244, "Session ID"=w243) -> ("error out"=w222:errorcluster, "Python Object References Out"=w224:T5, "Session ID out"=w226:T4)  [unwired: 5 in]
                n52 = call <vilib>:"Pack.vi"("Argument"=w220, "error in (no error)"=w222, "Python Object References In"=w224, "Session ID"=w226) -> ("error out"=w221:errorcluster, "Python Object References Out"=w223:T5, "Session ID out"=w225:T4)  [unwired: 5 in]
                n53 = call <vilib>:"Call.vi"("Function or Method Name"="PE_N_paramFive", "error in (no error)"=w221, "Python Object References In"=w223, "Session ID"=w225) -> ("error out"=w248:errorcluster, "Python Object References Out"=w251:T5, "Session ID out"=w254:T4)  [unwired: 5 in]
                n54 = call-poly <vilib>:"Unpack.vi"("error in (no error)"=w248, "Python Object References In"=w251, "Session ID"=w254) -> ("error out"=w238:errorcluster, "Value"=w236:dbl, "Python Object References Out"=w250:T5, "Session ID out"=w253:T4)  [unwired: 5 in]
                "Temp 2" <- w236
                n55 = call-poly <vilib>:"Unpack.vi"("error in (no error)"=w238, "Python Object References In"=w250, "Session ID"=w253) -> ("error out"=w247:errorcluster, "Value"=w235:dbl, "Python Object References Out"=w249:T5, "Session ID out"=w252:T4)  [unwired: 5 in]
                "Flow 2" <- w235
                n56 = call-poly <vilib>:"Unpack.vi"("error in (no error)"=w247, "Python Object References In"=w249, "Session ID"=w252) -> ("error out"=w237:errorcluster, "Value"=w234:dbl, "Python Object References Out"=w245:T5, "Session ID out"=w246:T4)  [unwired: 5 in]
                "Conc 2" <- w234
                n57 = call-poly <vilib>:"Unpack.vi"("error in (no error)"=w237, "Python Object References In"=w245, "Session ID"=w246) -> ("error out"=w267:errorcluster, "Value"=→"t1 - 1":dbl, "Python Object References Out"=w265:T5, "Session ID out"=w263:T4)  [unwired: 5 in]
                n58 = call-poly <vilib>:"Unpack.vi"("error in (no error)"=w267, "Python Object References In"=w265, "Session ID"=w263) -> ("error out"=w268:errorcluster, "Value"=→"X2 ref A 1":dbl, "Python Object References Out"=w266:T5, "Session ID out"=w264:T4)  [unwired: 5 in]
                n59 = call-poly <vilib>:"Unpack.vi"("error in (no error)"=w268, "Python Object References In"=w266, "Session ID"=w264) -> ("error out"=w269:errorcluster, "Value"=→"X2 B 1":dbl, "Python Object References Out"=w260:T5, "Session ID out"=w259:T4)  [unwired: 5 in]
                n60 = call-poly <vilib>:"Unpack.vi"("error in (no error)"=w269, "Python Object References In"=w260, "Session ID"=w259) -> ("error out"=w240:errorcluster, "Value"=→"X ref B 1":dbl, "Session ID out"=w241:T4)  [unwired: 5 in, 1 out]
                n61 = call <vilib>:"Close Session.vi"("error in (no error)"=w240, "Session ID"=w241) -> ()  [unwired: 9 in, 1 out]
              }
            }
            "Exp 2" <- TRUE
          }
          frame 3 {
            n62 = flat-sequence {
              tunnel: w277 -> [w288]
              tunnel: w273 -> [w281]
              tunnel: [w317] -> w276
              tunnel: [w316] -> w275
              tunnel: [w315] -> w274
              tunnel: w273 -> [w310]
              tunnel: w272 -> [w309]
              tunnel: w271 -> [w308]
              tunnel: w270 -> [w301]
              frame #0 {
                n63 = call <vilib>:"New Session.vi"("Path to Python Module (.py File)"=path "C:/Users/User/Documents/LabVIEW Data/2015 Projects/Combined/HPLCandAppendAmb.py") -> ("error out"=w297:errorcluster, "Session ID out"=w296:T4)  [unwired: 9 in]
                n64 = call <vilib>:"Pack.vi"("Argument"=w288, "error in (no error)"=w297, "Session ID"=w296) -> ("error out"=w283:errorcluster, "Python Object References Out"=w285:T5, "Session ID out"=w287:T4)  [unwired: 6 in]
                n65 = call <vilib>:"Pack.vi"("Argument"=w281, "error in (no error)"=w283, "Python Object References In"=w285, "Session ID"=w287) -> ("error out"=w282:errorcluster, "Python Object References Out"=w284:T5, "Session ID out"=w286:T4)  [unwired: 5 in]
                n66 = call <vilib>:"Call.vi"("Function or Method Name"="HPLC", "error in (no error)"=w282, "Python Object References In"=w284, "Session ID"=w286) -> ("error out"=w298:errorcluster, "Python Object References Out"=w289:T5, "Session ID out"=w290:T4)  [unwired: 5 in]
                n67 = call-poly <vilib>:"Unpack.vi"("error in (no error)"=w298, "Python Object References In"=w289, "Session ID"=w290) -> ("error out"=w299:errorcluster, "Value"=→"C BAcid 2":dbl, "Python Object References Out"=w294:T5, "Session ID out"=w293:T4)  [unwired: 5 in]
                n68 = call-poly <vilib>:"Unpack.vi"("error in (no error)"=w299, "Python Object References In"=w294, "Session ID"=w293) -> ("error out"=w300:errorcluster, "Value"=→"C EB 2":dbl, "Session ID out"=w295:T4)  [unwired: 5 in, 1 out]
                n69 = call <vilib>:"Close Session.vi"("error in (no error)"=w300, "Session ID"=w295) -> ()  [unwired: 9 in, 1 out]
              }
              frame #1 {
                n70 = call <vilib>:"New Session.vi"("Path to Python Module (.py File)"=path "C:/Users/User/Documents/LabVIEW Data/2015 Projects/Combined/Conor_PE_MBDoE_Amb_LabVIEW.py") -> ("error out"=w343:errorcluster, "Session ID out"=w342:T4)  [unwired: 9 in]
                n71 = call <vilib>:"Pack.vi"("Argument"=w310, "error in (no error)"=w343, "Session ID"=w342) -> ("error out"=w336:errorcluster, "Python Object References Out"=w337:T5, "Session ID out"=w338:T4)  [unwired: 6 in]
                n72 = call <vilib>:"Pack.vi"("Argument"=w309, "error in (no error)"=w336, "Python Object References In"=w337, "Session ID"=w338) -> ("error out"=w323:errorcluster, "Python Object References Out"=w325:T5, "Session ID out"=w324:T4)  [unwired: 5 in]
                n73 = call <vilib>:"Pack.vi"("Argument"=w308, "error in (no error)"=w323, "Python Object References In"=w325, "Session ID"=w324) -> ("error out"=w305:errorcluster, "Python Object References Out"=w306:T5, "Session ID out"=w307:T4)  [unwired: 5 in]
                n74 = call <vilib>:"Pack.vi"("Argument"=w301, "error in (no error)"=w305, "Python Object References In"=w306, "Session ID"=w307) -> ("error out"=w304:errorcluster, "Python Object References Out"=w303:T5, "Session ID out"=w302:T4)  [unwired: 5 in]
                n75 = call <vilib>:"Call.vi"("Function or Method Name"="PE_N_paramFive", "error in (no error)"=w304, "Python Object References In"=w303, "Session ID"=w302) -> ("error out"=w329:errorcluster, "Python Object References Out"=w332:T5, "Session ID out"=w335:T4)  [unwired: 5 in]
                n76 = call-poly <vilib>:"Unpack.vi"("error in (no error)"=w329, "Python Object References In"=w332, "Session ID"=w335) -> ("error out"=w319:errorcluster, "Value"=w317:dbl, "Python Object References Out"=w331:T5, "Session ID out"=w334:T4)  [unwired: 5 in]
                "Temp 3" <- w317
                n77 = call-poly <vilib>:"Unpack.vi"("error in (no error)"=w319, "Python Object References In"=w331, "Session ID"=w334) -> ("error out"=w328:errorcluster, "Value"=w316:dbl, "Python Object References Out"=w330:T5, "Session ID out"=w333:T4)  [unwired: 5 in]
                "Flow 3" <- w316
                n78 = call-poly <vilib>:"Unpack.vi"("error in (no error)"=w328, "Python Object References In"=w330, "Session ID"=w333) -> ("error out"=w318:errorcluster, "Value"=w315:dbl, "Python Object References Out"=w326:T5, "Session ID out"=w327:T4)  [unwired: 5 in]
                "Conc 3" <- w315
                n79 = call-poly <vilib>:"Unpack.vi"("error in (no error)"=w318, "Python Object References In"=w326, "Session ID"=w327) -> ("error out"=w348:errorcluster, "Value"=→"t1 2":dbl, "Python Object References Out"=w346:T5, "Session ID out"=w344:T4)  [unwired: 5 in]
                n80 = call-poly <vilib>:"Unpack.vi"("error in (no error)"=w348, "Python Object References In"=w346, "Session ID"=w344) -> ("error out"=w349:errorcluster, "Value"=→"X2 ref A 2":dbl, "Python Object References Out"=w347:T5, "Session ID out"=w345:T4)  [unwired: 5 in]
                n81 = call-poly <vilib>:"Unpack.vi"("error in (no error)"=w349, "Python Object References In"=w347, "Session ID"=w345) -> ("error out"=w350:errorcluster, "Value"=→"X2 B 2":dbl, "Python Object References Out"=w341:T5, "Session ID out"=w340:T4)  [unwired: 5 in]
                n82 = call-poly <vilib>:"Unpack.vi"("error in (no error)"=w350, "Python Object References In"=w341, "Session ID"=w340) -> ("error out"=w321:errorcluster, "Value"=→"X ref B 2":dbl, "Session ID out"=w322:T4)  [unwired: 5 in, 1 out]
                n83 = call <vilib>:"Close Session.vi"("error in (no error)"=w321, "Session ID"=w322) -> ()  [unwired: 9 in, 1 out]
              }
            }
            "Exp 3" <- TRUE
          }
          frame 4 {
            n84 = flat-sequence {
              tunnel: w358 -> [w369]
              tunnel: w354 -> [w362]
              tunnel: [w398] -> w357
              tunnel: [w397] -> w356
              tunnel: [w396] -> w355
              tunnel: w354 -> [w391]
              tunnel: w353 -> [w390]
              tunnel: w352 -> [w389]
              tunnel: w351 -> [w382]
              frame #0 {
                n85 = call <vilib>:"New Session.vi"("Path to Python Module (.py File)"=path "C:/Users/User/Documents/LabVIEW Data/2015 Projects/Combined/HPLCandAppendAmb.py") -> ("error out"=w378:errorcluster, "Session ID out"=w377:T4)  [unwired: 9 in]
                n86 = call <vilib>:"Pack.vi"("Argument"=w369, "error in (no error)"=w378, "Session ID"=w377) -> ("error out"=w364:errorcluster, "Python Object References Out"=w366:T5, "Session ID out"=w368:T4)  [unwired: 6 in]
                n87 = call <vilib>:"Pack.vi"("Argument"=w362, "error in (no error)"=w364, "Python Object References In"=w366, "Session ID"=w368) -> ("error out"=w363:errorcluster, "Python Object References Out"=w365:T5, "Session ID out"=w367:T4)  [unwired: 5 in]
                n88 = call <vilib>:"Call.vi"("Function or Method Name"="HPLC", "error in (no error)"=w363, "Python Object References In"=w365, "Session ID"=w367) -> ("error out"=w379:errorcluster, "Python Object References Out"=w370:T5, "Session ID out"=w371:T4)  [unwired: 5 in]
                n89 = call-poly <vilib>:"Unpack.vi"("error in (no error)"=w379, "Python Object References In"=w370, "Session ID"=w371) -> ("error out"=w380:errorcluster, "Value"=→"C BAcid 3":dbl, "Python Object References Out"=w375:T5, "Session ID out"=w374:T4)  [unwired: 5 in]
                n90 = call-poly <vilib>:"Unpack.vi"("error in (no error)"=w380, "Python Object References In"=w375, "Session ID"=w374) -> ("error out"=w381:errorcluster, "Value"=→"C EB 3":dbl, "Session ID out"=w376:T4)  [unwired: 5 in, 1 out]
                n91 = call <vilib>:"Close Session.vi"("error in (no error)"=w381, "Session ID"=w376) -> ()  [unwired: 9 in, 1 out]
              }
              frame #1 {
                n92 = call <vilib>:"New Session.vi"("Path to Python Module (.py File)"=path "C:/Users/User/Documents/LabVIEW Data/2015 Projects/Combined/Conor_PE_MBDoE_Amb_LabVIEW.py") -> ("error out"=w424:errorcluster, "Session ID out"=w423:T4)  [unwired: 9 in]
                n93 = call <vilib>:"Pack.vi"("Argument"=w391, "error in (no error)"=w424, "Session ID"=w423) -> ("error out"=w417:errorcluster, "Python Object References Out"=w418:T5, "Session ID out"=w419:T4)  [unwired: 6 in]
                n94 = call <vilib>:"Pack.vi"("Argument"=w390, "error in (no error)"=w417, "Python Object References In"=w418, "Session ID"=w419) -> ("error out"=w404:errorcluster, "Python Object References Out"=w406:T5, "Session ID out"=w405:T4)  [unwired: 5 in]
                n95 = call <vilib>:"Pack.vi"("Argument"=w389, "error in (no error)"=w404, "Python Object References In"=w406, "Session ID"=w405) -> ("error out"=w386:errorcluster, "Python Object References Out"=w387:T5, "Session ID out"=w388:T4)  [unwired: 5 in]
                n96 = call <vilib>:"Pack.vi"("Argument"=w382, "error in (no error)"=w386, "Python Object References In"=w387, "Session ID"=w388) -> ("error out"=w385:errorcluster, "Python Object References Out"=w384:T5, "Session ID out"=w383:T4)  [unwired: 5 in]
                n97 = call <vilib>:"Call.vi"("Function or Method Name"="PE_N_paramFive", "error in (no error)"=w385, "Python Object References In"=w384, "Session ID"=w383) -> ("error out"=w410:errorcluster, "Python Object References Out"=w413:T5, "Session ID out"=w416:T4)  [unwired: 5 in]
                n98 = call-poly <vilib>:"Unpack.vi"("error in (no error)"=w410, "Python Object References In"=w413, "Session ID"=w416) -> ("error out"=w400:errorcluster, "Value"=w398:dbl, "Python Object References Out"=w412:T5, "Session ID out"=w415:T4)  [unwired: 5 in]
                "Temp 4" <- w398
                n99 = call-poly <vilib>:"Unpack.vi"("error in (no error)"=w400, "Python Object References In"=w412, "Session ID"=w415) -> ("error out"=w409:errorcluster, "Value"=w397:dbl, "Python Object References Out"=w411:T5, "Session ID out"=w414:T4)  [unwired: 5 in]
                "Flow 4" <- w397
                n100 = call-poly <vilib>:"Unpack.vi"("error in (no error)"=w409, "Python Object References In"=w411, "Session ID"=w414) -> ("error out"=w399:errorcluster, "Value"=w396:dbl, "Python Object References Out"=w407:T5, "Session ID out"=w408:T4)  [unwired: 5 in]
                "Conc 4" <- w396
                n101 = call-poly <vilib>:"Unpack.vi"("error in (no error)"=w399, "Python Object References In"=w407, "Session ID"=w408) -> ("error out"=w429:errorcluster, "Value"=→"t1 - 3":dbl, "Python Object References Out"=w427:T5, "Session ID out"=w425:T4)  [unwired: 5 in]
                n102 = call-poly <vilib>:"Unpack.vi"("error in (no error)"=w429, "Python Object References In"=w427, "Session ID"=w425) -> ("error out"=w430:errorcluster, "Value"=→"X2 ref A 3":dbl, "Python Object References Out"=w428:T5, "Session ID out"=w426:T4)  [unwired: 5 in]
                n103 = call-poly <vilib>:"Unpack.vi"("error in (no error)"=w430, "Python Object References In"=w428, "Session ID"=w426) -> ("error out"=w431:errorcluster, "Value"=→"X2 B 3":dbl, "Python Object References Out"=w422:T5, "Session ID out"=w421:T4)  [unwired: 5 in]
                n104 = call-poly <vilib>:"Unpack.vi"("error in (no error)"=w431, "Python Object References In"=w422, "Session ID"=w421) -> ("error out"=w402:errorcluster, "Value"=→"X ref B 3":dbl, "Session ID out"=w403:T4)  [unwired: 5 in, 1 out]
                n105 = call <vilib>:"Close Session.vi"("error in (no error)"=w402, "Session ID"=w403) -> ()  [unwired: 9 in, 1 out]
              }
            }
            "Exp 4" <- TRUE
          }
          frame 5 {
            n106 = flat-sequence {
              tunnel: w439 -> [w450]
              tunnel: w435 -> [w443]
              tunnel: [w479] -> w438
              tunnel: [w478] -> w437
              tunnel: [w477] -> w436
              tunnel: w435 -> [w472]
              tunnel: w434 -> [w471]
              tunnel: w433 -> [w470]
              tunnel: w432 -> [w463]
              frame #0 {
                n107 = call <vilib>:"New Session.vi"("Path to Python Module (.py File)"=path "C:/Users/User/Documents/LabVIEW Data/2015 Projects/Combined/HPLCandAppendAmb.py") -> ("error out"=w459:errorcluster, "Session ID out"=w458:T4)  [unwired: 9 in]
                n108 = call <vilib>:"Pack.vi"("Argument"=w450, "error in (no error)"=w459, "Session ID"=w458) -> ("error out"=w445:errorcluster, "Python Object References Out"=w447:T5, "Session ID out"=w449:T4)  [unwired: 6 in]
                n109 = call <vilib>:"Pack.vi"("Argument"=w443, "error in (no error)"=w445, "Python Object References In"=w447, "Session ID"=w449) -> ("error out"=w444:errorcluster, "Python Object References Out"=w446:T5, "Session ID out"=w448:T4)  [unwired: 5 in]
                n110 = call <vilib>:"Call.vi"("Function or Method Name"="HPLC", "error in (no error)"=w444, "Python Object References In"=w446, "Session ID"=w448) -> ("error out"=w460:errorcluster, "Python Object References Out"=w451:T5, "Session ID out"=w452:T4)  [unwired: 5 in]
                n111 = call-poly <vilib>:"Unpack.vi"("error in (no error)"=w460, "Python Object References In"=w451, "Session ID"=w452) -> ("error out"=w461:errorcluster, "Value"=→"C BAcid 4":dbl, "Python Object References Out"=w456:T5, "Session ID out"=w455:T4)  [unwired: 5 in]
                n112 = call-poly <vilib>:"Unpack.vi"("error in (no error)"=w461, "Python Object References In"=w456, "Session ID"=w455) -> ("error out"=w462:errorcluster, "Value"=→"C EB 4":dbl, "Session ID out"=w457:T4)  [unwired: 5 in, 1 out]
                n113 = call <vilib>:"Close Session.vi"("error in (no error)"=w462, "Session ID"=w457) -> ()  [unwired: 9 in, 1 out]
              }
              frame #1 {
                n114 = call <vilib>:"New Session.vi"("Path to Python Module (.py File)"=path "C:/Users/User/Documents/LabVIEW Data/2015 Projects/Combined/Conor_PE_MBDoE_Amb_LabVIEW.py") -> ("error out"=w505:errorcluster, "Session ID out"=w504:T4)  [unwired: 9 in]
                n115 = call <vilib>:"Pack.vi"("Argument"=w472, "error in (no error)"=w505, "Session ID"=w504) -> ("error out"=w498:errorcluster, "Python Object References Out"=w499:T5, "Session ID out"=w500:T4)  [unwired: 6 in]
                n116 = call <vilib>:"Pack.vi"("Argument"=w471, "error in (no error)"=w498, "Python Object References In"=w499, "Session ID"=w500) -> ("error out"=w485:errorcluster, "Python Object References Out"=w487:T5, "Session ID out"=w486:T4)  [unwired: 5 in]
                n117 = call <vilib>:"Pack.vi"("Argument"=w470, "error in (no error)"=w485, "Python Object References In"=w487, "Session ID"=w486) -> ("error out"=w465:errorcluster, "Python Object References Out"=w467:T5, "Session ID out"=w469:T4)  [unwired: 5 in]
                n118 = call <vilib>:"Pack.vi"("Argument"=w463, "error in (no error)"=w465, "Python Object References In"=w467, "Session ID"=w469) -> ("error out"=w464:errorcluster, "Python Object References Out"=w466:T5, "Session ID out"=w468:T4)  [unwired: 5 in]
                n119 = call <vilib>:"Call.vi"("Function or Method Name"="PE_N_paramFive", "error in (no error)"=w464, "Python Object References In"=w466, "Session ID"=w468) -> ("error out"=w491:errorcluster, "Python Object References Out"=w494:T5, "Session ID out"=w497:T4)  [unwired: 5 in]
                n120 = call-poly <vilib>:"Unpack.vi"("error in (no error)"=w491, "Python Object References In"=w494, "Session ID"=w497) -> ("error out"=w481:errorcluster, "Value"=w479:dbl, "Python Object References Out"=w493:T5, "Session ID out"=w496:T4)  [unwired: 5 in]
                "Temp 5" <- w479
                n121 = call-poly <vilib>:"Unpack.vi"("error in (no error)"=w481, "Python Object References In"=w493, "Session ID"=w496) -> ("error out"=w490:errorcluster, "Value"=w478:dbl, "Python Object References Out"=w492:T5, "Session ID out"=w495:T4)  [unwired: 5 in]
                "Flow 5" <- w478
                n122 = call-poly <vilib>:"Unpack.vi"("error in (no error)"=w490, "Python Object References In"=w492, "Session ID"=w495) -> ("error out"=w480:errorcluster, "Value"=w477:dbl, "Python Object References Out"=w488:T5, "Session ID out"=w489:T4)  [unwired: 5 in]
                "Conc 5" <- w477
                n123 = call-poly <vilib>:"Unpack.vi"("error in (no error)"=w480, "Python Object References In"=w488, "Session ID"=w489) -> ("error out"=w510:errorcluster, "Value"=→"t1 - 4":dbl, "Python Object References Out"=w508:T5, "Session ID out"=w506:T4)  [unwired: 5 in]
                n124 = call-poly <vilib>:"Unpack.vi"("error in (no error)"=w510, "Python Object References In"=w508, "Session ID"=w506) -> ("error out"=w511:errorcluster, "Value"=→"X2 ref A 4":dbl, "Python Object References Out"=w509:T5, "Session ID out"=w507:T4)  [unwired: 5 in]
                n125 = call-poly <vilib>:"Unpack.vi"("error in (no error)"=w511, "Python Object References In"=w509, "Session ID"=w507) -> ("error out"=w512:errorcluster, "Value"=→"X2 B 4":dbl, "Python Object References Out"=w503:T5, "Session ID out"=w502:T4)  [unwired: 5 in]
                n126 = call-poly <vilib>:"Unpack.vi"("error in (no error)"=w512, "Python Object References In"=w503, "Session ID"=w502) -> ("error out"=w483:errorcluster, "Value"=→"X ref B 4":dbl, "Session ID out"=w484:T4)  [unwired: 5 in, 1 out]
                n127 = call <vilib>:"Close Session.vi"("error in (no error)"=w483, "Session ID"=w484) -> ()  [unwired: 9 in, 1 out]
              }
            }
            "Exp 5" <- TRUE
          }
          frame 6 {
            n128 = flat-sequence {
              tunnel: w520 -> [w531]
              tunnel: w516 -> [w524]
              tunnel: [w560] -> w519
              tunnel: [w559] -> w518
              tunnel: [w558] -> w517
              tunnel: w516 -> [w553]
              tunnel: w515 -> [w552]
              tunnel: w514 -> [w551]
              tunnel: w513 -> [w544]
              frame #0 {
                n129 = call <vilib>:"New Session.vi"("Path to Python Module (.py File)"=path "C:/Users/User/Documents/LabVIEW Data/2015 Projects/Combined/HPLCandAppendAmb.py") -> ("error out"=w540:errorcluster, "Session ID out"=w539:T4)  [unwired: 9 in]
                n130 = call <vilib>:"Pack.vi"("Argument"=w531, "error in (no error)"=w540, "Session ID"=w539) -> ("error out"=w526:errorcluster, "Python Object References Out"=w528:T5, "Session ID out"=w530:T4)  [unwired: 6 in]
                n131 = call <vilib>:"Pack.vi"("Argument"=w524, "error in (no error)"=w526, "Python Object References In"=w528, "Session ID"=w530) -> ("error out"=w525:errorcluster, "Python Object References Out"=w527:T5, "Session ID out"=w529:T4)  [unwired: 5 in]
                n132 = call <vilib>:"Call.vi"("Function or Method Name"="HPLC", "error in (no error)"=w525, "Python Object References In"=w527, "Session ID"=w529) -> ("error out"=w541:errorcluster, "Python Object References Out"=w532:T5, "Session ID out"=w533:T4)  [unwired: 5 in]
                n133 = call-poly <vilib>:"Unpack.vi"("error in (no error)"=w541, "Python Object References In"=w532, "Session ID"=w533) -> ("error out"=w542:errorcluster, "Value"=→"C BAcid 5":dbl, "Python Object References Out"=w537:T5, "Session ID out"=w536:T4)  [unwired: 5 in]
                n134 = call-poly <vilib>:"Unpack.vi"("error in (no error)"=w542, "Python Object References In"=w537, "Session ID"=w536) -> ("error out"=w543:errorcluster, "Value"=→"C EB 5":dbl, "Session ID out"=w538:T4)  [unwired: 5 in, 1 out]
                n135 = call <vilib>:"Close Session.vi"("error in (no error)"=w543, "Session ID"=w538) -> ()  [unwired: 9 in, 1 out]
              }
              frame #1 {
                n136 = call <vilib>:"New Session.vi"("Path to Python Module (.py File)"=path "C:/Users/User/Documents/LabVIEW Data/2015 Projects/Combined/Conor_PE_MBDoE_Amb_LabVIEW.py") -> ("error out"=w586:errorcluster, "Session ID out"=w585:T4)  [unwired: 9 in]
                n137 = call <vilib>:"Pack.vi"("Argument"=w553, "error in (no error)"=w586, "Session ID"=w585) -> ("error out"=w579:errorcluster, "Python Object References Out"=w580:T5, "Session ID out"=w581:T4)  [unwired: 6 in]
                n138 = call <vilib>:"Pack.vi"("Argument"=w552, "error in (no error)"=w579, "Python Object References In"=w580, "Session ID"=w581) -> ("error out"=w566:errorcluster, "Python Object References Out"=w568:T5, "Session ID out"=w567:T4)  [unwired: 5 in]
                n139 = call <vilib>:"Pack.vi"("Argument"=w551, "error in (no error)"=w566, "Python Object References In"=w568, "Session ID"=w567) -> ("error out"=w546:errorcluster, "Python Object References Out"=w548:T5, "Session ID out"=w550:T4)  [unwired: 5 in]
                n140 = call <vilib>:"Pack.vi"("Argument"=w544, "error in (no error)"=w546, "Python Object References In"=w548, "Session ID"=w550) -> ("error out"=w545:errorcluster, "Python Object References Out"=w547:T5, "Session ID out"=w549:T4)  [unwired: 5 in]
                n141 = call <vilib>:"Call.vi"("Function or Method Name"="PE_N_paramFive", "error in (no error)"=w545, "Python Object References In"=w547, "Session ID"=w549) -> ("error out"=w572:errorcluster, "Python Object References Out"=w575:T5, "Session ID out"=w578:T4)  [unwired: 5 in]
                n142 = call-poly <vilib>:"Unpack.vi"("error in (no error)"=w572, "Python Object References In"=w575, "Session ID"=w578) -> ("error out"=w562:errorcluster, "Value"=w560:dbl, "Python Object References Out"=w574:T5, "Session ID out"=w577:T4)  [unwired: 5 in]
                "Temp 6" <- w560
                n143 = call-poly <vilib>:"Unpack.vi"("error in (no error)"=w562, "Python Object References In"=w574, "Session ID"=w577) -> ("error out"=w571:errorcluster, "Value"=w559:dbl, "Python Object References Out"=w573:T5, "Session ID out"=w576:T4)  [unwired: 5 in]
                "Flow 6" <- w559
                n144 = call-poly <vilib>:"Unpack.vi"("error in (no error)"=w571, "Python Object References In"=w573, "Session ID"=w576) -> ("error out"=w561:errorcluster, "Value"=w558:dbl, "Python Object References Out"=w569:T5, "Session ID out"=w570:T4)  [unwired: 5 in]
                "Conc 6" <- w558
                n145 = call-poly <vilib>:"Unpack.vi"("error in (no error)"=w561, "Python Object References In"=w569, "Session ID"=w570) -> ("error out"=w591:errorcluster, "Value"=→"t1 - 5":dbl, "Python Object References Out"=w589:T5, "Session ID out"=w587:T4)  [unwired: 5 in]
                n146 = call-poly <vilib>:"Unpack.vi"("error in (no error)"=w591, "Python Object References In"=w589, "Session ID"=w587) -> ("error out"=w592:errorcluster, "Value"=→"X2 ref A 5":dbl, "Python Object References Out"=w590:T5, "Session ID out"=w588:T4)  [unwired: 5 in]
                n147 = call-poly <vilib>:"Unpack.vi"("error in (no error)"=w592, "Python Object References In"=w590, "Session ID"=w588) -> ("error out"=w593:errorcluster, "Value"=→"X2 B 5":dbl, "Python Object References Out"=w584:T5, "Session ID out"=w583:T4)  [unwired: 5 in]
                n148 = call-poly <vilib>:"Unpack.vi"("error in (no error)"=w593, "Python Object References In"=w584, "Session ID"=w583) -> ("error out"=w564:errorcluster, "Value"=→"X ref B 5":dbl, "Session ID out"=w565:T4)  [unwired: 5 in, 1 out]
                n149 = call <vilib>:"Close Session.vi"("error in (no error)"=w564, "Session ID"=w565) -> ()  [unwired: 9 in, 1 out]
              }
            }
            "Exp 6" <- TRUE
          }
          frame 7 {
            n150 = flat-sequence {
              tunnel: w601 -> [w612]
              tunnel: w597 -> [w605]
              tunnel: [w641] -> w600
              tunnel: [w640] -> w599
              tunnel: [w639] -> w598
              tunnel: w597 -> [w634]
              tunnel: w596 -> [w633]
              tunnel: w595 -> [w632]
              tunnel: w594 -> [w625]
              frame #0 {
                n151 = call <vilib>:"New Session.vi"("Path to Python Module (.py File)"=path "C:/Users/User/Documents/LabVIEW Data/2015 Projects/Combined/HPLCandAppendAmb.py") -> ("error out"=w621:errorcluster, "Session ID out"=w620:T4)  [unwired: 9 in]
                n152 = call <vilib>:"Pack.vi"("Argument"=w612, "error in (no error)"=w621, "Session ID"=w620) -> ("error out"=w607:errorcluster, "Python Object References Out"=w609:T5, "Session ID out"=w611:T4)  [unwired: 6 in]
                n153 = call <vilib>:"Pack.vi"("Argument"=w605, "error in (no error)"=w607, "Python Object References In"=w609, "Session ID"=w611) -> ("error out"=w606:errorcluster, "Python Object References Out"=w608:T5, "Session ID out"=w610:T4)  [unwired: 5 in]
                n154 = call <vilib>:"Call.vi"("Function or Method Name"="HPLC", "error in (no error)"=w606, "Python Object References In"=w608, "Session ID"=w610) -> ("error out"=w622:errorcluster, "Python Object References Out"=w613:T5, "Session ID out"=w614:T4)  [unwired: 5 in]
                n155 = call-poly <vilib>:"Unpack.vi"("error in (no error)"=w622, "Python Object References In"=w613, "Session ID"=w614) -> ("error out"=w623:errorcluster, "Value"=→"C BAcid 6":dbl, "Python Object References Out"=w618:T5, "Session ID out"=w617:T4)  [unwired: 5 in]
                n156 = call-poly <vilib>:"Unpack.vi"("error in (no error)"=w623, "Python Object References In"=w618, "Session ID"=w617) -> ("error out"=w624:errorcluster, "Value"=→"C EB 6":dbl, "Session ID out"=w619:T4)  [unwired: 5 in, 1 out]
                n157 = call <vilib>:"Close Session.vi"("error in (no error)"=w624, "Session ID"=w619) -> ()  [unwired: 9 in, 1 out]
              }
              frame #1 {
                n158 = call <vilib>:"New Session.vi"("Path to Python Module (.py File)"=path "C:/Users/User/Documents/LabVIEW Data/2015 Projects/Combined/Conor_PE_MBDoE_Amb_LabVIEW.py") -> ("error out"=w667:errorcluster, "Session ID out"=w666:T4)  [unwired: 9 in]
                n159 = call <vilib>:"Pack.vi"("Argument"=w634, "error in (no error)"=w667, "Session ID"=w666) -> ("error out"=w660:errorcluster, "Python Object References Out"=w661:T5, "Session ID out"=w662:T4)  [unwired: 6 in]
                n160 = call <vilib>:"Pack.vi"("Argument"=w633, "error in (no error)"=w660, "Python Object References In"=w661, "Session ID"=w662) -> ("error out"=w647:errorcluster, "Python Object References Out"=w649:T5, "Session ID out"=w648:T4)  [unwired: 5 in]
                n161 = call <vilib>:"Pack.vi"("Argument"=w632, "error in (no error)"=w647, "Python Object References In"=w649, "Session ID"=w648) -> ("error out"=w627:errorcluster, "Python Object References Out"=w629:T5, "Session ID out"=w631:T4)  [unwired: 5 in]
                n162 = call <vilib>:"Pack.vi"("Argument"=w625, "error in (no error)"=w627, "Python Object References In"=w629, "Session ID"=w631) -> ("error out"=w626:errorcluster, "Python Object References Out"=w628:T5, "Session ID out"=w630:T4)  [unwired: 5 in]
                n163 = call <vilib>:"Call.vi"("Function or Method Name"="PE_N_paramFive", "error in (no error)"=w626, "Python Object References In"=w628, "Session ID"=w630) -> ("error out"=w653:errorcluster, "Python Object References Out"=w656:T5, "Session ID out"=w659:T4)  [unwired: 5 in]
                n164 = call-poly <vilib>:"Unpack.vi"("error in (no error)"=w653, "Python Object References In"=w656, "Session ID"=w659) -> ("error out"=w643:errorcluster, "Value"=w641:dbl, "Python Object References Out"=w655:T5, "Session ID out"=w658:T4)  [unwired: 5 in]
                "Temp 7" <- w641
                n165 = call-poly <vilib>:"Unpack.vi"("error in (no error)"=w643, "Python Object References In"=w655, "Session ID"=w658) -> ("error out"=w652:errorcluster, "Value"=w640:dbl, "Python Object References Out"=w654:T5, "Session ID out"=w657:T4)  [unwired: 5 in]
                "Flow 7" <- w640
                n166 = call-poly <vilib>:"Unpack.vi"("error in (no error)"=w652, "Python Object References In"=w654, "Session ID"=w657) -> ("error out"=w642:errorcluster, "Value"=w639:dbl, "Python Object References Out"=w650:T5, "Session ID out"=w651:T4)  [unwired: 5 in]
                "Conc 7" <- w639
                n167 = call-poly <vilib>:"Unpack.vi"("error in (no error)"=w642, "Python Object References In"=w650, "Session ID"=w651) -> ("error out"=w672:errorcluster, "Value"=→"t1 - 6":dbl, "Python Object References Out"=w670:T5, "Session ID out"=w668:T4)  [unwired: 5 in]
                n168 = call-poly <vilib>:"Unpack.vi"("error in (no error)"=w672, "Python Object References In"=w670, "Session ID"=w668) -> ("error out"=w673:errorcluster, "Value"=→"X2 ref A 6":dbl, "Python Object References Out"=w671:T5, "Session ID out"=w669:T4)  [unwired: 5 in]
                n169 = call-poly <vilib>:"Unpack.vi"("error in (no error)"=w673, "Python Object References In"=w671, "Session ID"=w669) -> ("error out"=w674:errorcluster, "Value"=→"X2 B 6":dbl, "Python Object References Out"=w665:T5, "Session ID out"=w664:T4)  [unwired: 5 in]
                n170 = call-poly <vilib>:"Unpack.vi"("error in (no error)"=w674, "Python Object References In"=w665, "Session ID"=w664) -> ("error out"=w645:errorcluster, "Value"=→"X ref B 6":dbl, "Session ID out"=w646:T4)  [unwired: 5 in, 1 out]
                n171 = call <vilib>:"Close Session.vi"("error in (no error)"=w645, "Session ID"=w646) -> ()  [unwired: 9 in, 1 out]
              }
            }
            "Exp 7" <- TRUE
          }
          frame 8 {
            n172 = flat-sequence {
              tunnel: w682 -> [w693]
              tunnel: w678 -> [w686]
              tunnel: [w722] -> w681
              tunnel: [w721] -> w680
              tunnel: [w720] -> w679
              tunnel: w678 -> [w715]
              tunnel: w677 -> [w714]
              tunnel: w676 -> [w713]
              tunnel: w675 -> [w706]
              frame #0 {
                n173 = call <vilib>:"New Session.vi"("Path to Python Module (.py File)"=path "C:/Users/User/Documents/LabVIEW Data/2015 Projects/Combined/HPLCandAppendAmb.py") -> ("error out"=w702:errorcluster, "Session ID out"=w701:T4)  [unwired: 9 in]
                n174 = call <vilib>:"Pack.vi"("Argument"=w693, "error in (no error)"=w702, "Session ID"=w701) -> ("error out"=w688:errorcluster, "Python Object References Out"=w690:T5, "Session ID out"=w692:T4)  [unwired: 6 in]
                n175 = call <vilib>:"Pack.vi"("Argument"=w686, "error in (no error)"=w688, "Python Object References In"=w690, "Session ID"=w692) -> ("error out"=w687:errorcluster, "Python Object References Out"=w689:T5, "Session ID out"=w691:T4)  [unwired: 5 in]
                n176 = call <vilib>:"Call.vi"("Function or Method Name"="HPLC", "error in (no error)"=w687, "Python Object References In"=w689, "Session ID"=w691) -> ("error out"=w703:errorcluster, "Python Object References Out"=w694:T5, "Session ID out"=w695:T4)  [unwired: 5 in]
                n177 = call-poly <vilib>:"Unpack.vi"("error in (no error)"=w703, "Python Object References In"=w694, "Session ID"=w695) -> ("error out"=w704:errorcluster, "Value"=→"C BAcid 7":dbl, "Python Object References Out"=w699:T5, "Session ID out"=w698:T4)  [unwired: 5 in]
                n178 = call-poly <vilib>:"Unpack.vi"("error in (no error)"=w704, "Python Object References In"=w699, "Session ID"=w698) -> ("error out"=w705:errorcluster, "Value"=→"C EB 7":dbl, "Session ID out"=w700:T4)  [unwired: 5 in, 1 out]
                n179 = call <vilib>:"Close Session.vi"("error in (no error)"=w705, "Session ID"=w700) -> ()  [unwired: 9 in, 1 out]
              }
              frame #1 {
                n180 = call <vilib>:"New Session.vi"("Path to Python Module (.py File)"=path "C:/Users/User/Documents/LabVIEW Data/2015 Projects/Combined/Conor_PE_MBDoE_Amb_LabVIEW.py") -> ("error out"=w748:errorcluster, "Session ID out"=w747:T4)  [unwired: 9 in]
                n181 = call <vilib>:"Pack.vi"("Argument"=w715, "error in (no error)"=w748, "Session ID"=w747) -> ("error out"=w741:errorcluster, "Python Object References Out"=w742:T5, "Session ID out"=w743:T4)  [unwired: 6 in]
                n182 = call <vilib>:"Pack.vi"("Argument"=w714, "error in (no error)"=w741, "Python Object References In"=w742, "Session ID"=w743) -> ("error out"=w728:errorcluster, "Python Object References Out"=w730:T5, "Session ID out"=w729:T4)  [unwired: 5 in]
                n183 = call <vilib>:"Pack.vi"("Argument"=w713, "error in (no error)"=w728, "Python Object References In"=w730, "Session ID"=w729) -> ("error out"=w708:errorcluster, "Python Object References Out"=w710:T5, "Session ID out"=w712:T4)  [unwired: 5 in]
                n184 = call <vilib>:"Pack.vi"("Argument"=w706, "error in (no error)"=w708, "Python Object References In"=w710, "Session ID"=w712) -> ("error out"=w707:errorcluster, "Python Object References Out"=w709:T5, "Session ID out"=w711:T4)  [unwired: 5 in]
                n185 = call <vilib>:"Call.vi"("Function or Method Name"="PE_N_paramFive", "error in (no error)"=w707, "Python Object References In"=w709, "Session ID"=w711) -> ("error out"=w734:errorcluster, "Python Object References Out"=w737:T5, "Session ID out"=w740:T4)  [unwired: 5 in]
                n186 = call-poly <vilib>:"Unpack.vi"("error in (no error)"=w734, "Python Object References In"=w737, "Session ID"=w740) -> ("error out"=w724:errorcluster, "Value"=w722:dbl, "Python Object References Out"=w736:T5, "Session ID out"=w739:T4)  [unwired: 5 in]
                "Temp 8" <- w722
                n187 = call-poly <vilib>:"Unpack.vi"("error in (no error)"=w724, "Python Object References In"=w736, "Session ID"=w739) -> ("error out"=w733:errorcluster, "Value"=w721:dbl, "Python Object References Out"=w735:T5, "Session ID out"=w738:T4)  [unwired: 5 in]
                "Flow 8" <- w721
                n188 = call-poly <vilib>:"Unpack.vi"("error in (no error)"=w733, "Python Object References In"=w735, "Session ID"=w738) -> ("error out"=w723:errorcluster, "Value"=w720:dbl, "Python Object References Out"=w731:T5, "Session ID out"=w732:T4)  [unwired: 5 in]
                "Conc 8" <- w720
                n189 = call-poly <vilib>:"Unpack.vi"("error in (no error)"=w723, "Python Object References In"=w731, "Session ID"=w732) -> ("error out"=w753:errorcluster, "Value"=→"t1 - 7":dbl, "Python Object References Out"=w751:T5, "Session ID out"=w749:T4)  [unwired: 5 in]
                n190 = call-poly <vilib>:"Unpack.vi"("error in (no error)"=w753, "Python Object References In"=w751, "Session ID"=w749) -> ("error out"=w754:errorcluster, "Value"=→"X2 ref A 7":dbl, "Python Object References Out"=w752:T5, "Session ID out"=w750:T4)  [unwired: 5 in]
                n191 = call-poly <vilib>:"Unpack.vi"("error in (no error)"=w754, "Python Object References In"=w752, "Session ID"=w750) -> ("error out"=w755:errorcluster, "Value"=→"X2 B 7":dbl, "Python Object References Out"=w746:T5, "Session ID out"=w745:T4)  [unwired: 5 in]
                n192 = call-poly <vilib>:"Unpack.vi"("error in (no error)"=w755, "Python Object References In"=w746, "Session ID"=w745) -> ("error out"=w726:errorcluster, "Value"=→"X ref B 7":dbl, "Session ID out"=w727:T4)  [unwired: 5 in, 1 out]
                n193 = call <vilib>:"Close Session.vi"("error in (no error)"=w726, "Session ID"=w727) -> ()  [unwired: 9 in, 1 out]
              }
            }
            "Exp 8" <- TRUE
          }
          frame 9 {
            n194 = flat-sequence {
              tunnel: w763 -> [w774]
              tunnel: w759 -> [w767]
              tunnel: w759 -> [w796]
              tunnel: w758 -> [w795]
              tunnel: w757 -> [w794]
              tunnel: w756 -> [w787]
              frame #0 {
                n195 = call <vilib>:"New Session.vi"("Path to Python Module (.py File)"=path "C:/Users/User/Documents/LabVIEW Data/2015 Projects/Combined/HPLCandAppendAmb.py") -> ("error out"=w783:errorcluster, "Session ID out"=w782:T4)  [unwired: 9 in]
                n196 = call <vilib>:"Pack.vi"("Argument"=w774, "error in (no error)"=w783, "Session ID"=w782) -> ("error out"=w769:errorcluster, "Python Object References Out"=w771:T5, "Session ID out"=w773:T4)  [unwired: 6 in]
                n197 = call <vilib>:"Pack.vi"("Argument"=w767, "error in (no error)"=w769, "Python Object References In"=w771, "Session ID"=w773) -> ("error out"=w768:errorcluster, "Python Object References Out"=w770:T5, "Session ID out"=w772:T4)  [unwired: 5 in]
                n198 = call <vilib>:"Call.vi"("Function or Method Name"="HPLC", "error in (no error)"=w768, "Python Object References In"=w770, "Session ID"=w772) -> ("error out"=w784:errorcluster, "Python Object References Out"=w775:T5, "Session ID out"=w776:T4)  [unwired: 5 in]
                n199 = call-poly <vilib>:"Unpack.vi"("error in (no error)"=w784, "Python Object References In"=w775, "Session ID"=w776) -> ("error out"=w785:errorcluster, "Value"=→"C BAcid 8":dbl, "Python Object References Out"=w780:T5, "Session ID out"=w779:T4)  [unwired: 5 in]
                n200 = call-poly <vilib>:"Unpack.vi"("error in (no error)"=w785, "Python Object References In"=w780, "Session ID"=w779) -> ("error out"=w786:errorcluster, "Value"=→"C EB 8":dbl, "Session ID out"=w781:T4)  [unwired: 5 in, 1 out]
                n201 = call <vilib>:"Close Session.vi"("error in (no error)"=w786, "Session ID"=w781) -> ()  [unwired: 9 in, 1 out]
              }
              frame #1 {
                n202 = call <vilib>:"New Session.vi"("Path to Python Module (.py File)"=path "C:/Users/User/Documents/LabVIEW Data/2015 Projects/Combined/Conor_PE_MBDoE_Amb_LabVIEW.py") -> ("error out"=w829:errorcluster, "Session ID out"=w828:T4)  [unwired: 9 in]
                n203 = call <vilib>:"Pack.vi"("Argument"=w796, "error in (no error)"=w829, "Session ID"=w828) -> ("error out"=w822:errorcluster, "Python Object References Out"=w823:T5, "Session ID out"=w824:T4)  [unwired: 6 in]
                n204 = call <vilib>:"Pack.vi"("Argument"=w795, "error in (no error)"=w822, "Python Object References In"=w823, "Session ID"=w824) -> ("error out"=w809:errorcluster, "Python Object References Out"=w811:T5, "Session ID out"=w810:T4)  [unwired: 5 in]
                n205 = call <vilib>:"Pack.vi"("Argument"=w794, "error in (no error)"=w809, "Python Object References In"=w811, "Session ID"=w810) -> ("error out"=w789:errorcluster, "Python Object References Out"=w791:T5, "Session ID out"=w793:T4)  [unwired: 5 in]
                n206 = call <vilib>:"Pack.vi"("Argument"=w787, "error in (no error)"=w789, "Python Object References In"=w791, "Session ID"=w793) -> ("error out"=w788:errorcluster, "Python Object References Out"=w790:T5, "Session ID out"=w792:T4)  [unwired: 5 in]
                n207 = call <vilib>:"Call.vi"("Function or Method Name"="PE_N_paramFive", "error in (no error)"=w788, "Python Object References In"=w790, "Session ID"=w792) -> ("error out"=w815:errorcluster, "Python Object References Out"=w818:T5, "Session ID out"=w821:T4)  [unwired: 5 in]
                n208 = call-poly <vilib>:"Unpack.vi"("error in (no error)"=w815, "Python Object References In"=w818, "Session ID"=w821) -> ("error out"=w805:errorcluster, "Value"=→"Temp 9":dbl, "Python Object References Out"=w817:T5, "Session ID out"=w820:T4)  [unwired: 5 in]
                n209 = call-poly <vilib>:"Unpack.vi"("error in (no error)"=w805, "Python Object References In"=w817, "Session ID"=w820) -> ("error out"=w814:errorcluster, "Value"=→"Flow 9":dbl, "Python Object References Out"=w816:T5, "Session ID out"=w819:T4)  [unwired: 5 in]
                n210 = call-poly <vilib>:"Unpack.vi"("error in (no error)"=w814, "Python Object References In"=w816, "Session ID"=w819) -> ("error out"=w804:errorcluster, "Value"=→"Conc 9":dbl, "Python Object References Out"=w812:T5, "Session ID out"=w813:T4)  [unwired: 5 in]
                n211 = call-poly <vilib>:"Unpack.vi"("error in (no error)"=w804, "Python Object References In"=w812, "Session ID"=w813) -> ("error out"=w834:errorcluster, "Value"=→"t1 - 8":dbl, "Python Object References Out"=w832:T5, "Session ID out"=w830:T4)  [unwired: 5 in]
                n212 = call-poly <vilib>:"Unpack.vi"("error in (no error)"=w834, "Python Object References In"=w832, "Session ID"=w830) -> ("error out"=w835:errorcluster, "Value"=→"X2 ref A 8":dbl, "Python Object References Out"=w833:T5, "Session ID out"=w831:T4)  [unwired: 5 in]
                n213 = call-poly <vilib>:"Unpack.vi"("error in (no error)"=w835, "Python Object References In"=w833, "Session ID"=w831) -> ("error out"=w836:errorcluster, "Value"=→"X2 B 8":dbl, "Python Object References Out"=w827:T5, "Session ID out"=w826:T4)  [unwired: 5 in]
                n214 = call-poly <vilib>:"Unpack.vi"("error in (no error)"=w836, "Python Object References In"=w827, "Session ID"=w826) -> ("error out"=w807:errorcluster, "Value"=→"X ref B 8":dbl, "Session ID out"=w808:T4)  [unwired: 5 in, 1 out]
                n215 = call <vilib>:"Close Session.vi"("error in (no error)"=w807, "Session ID"=w808) -> ()  [unwired: 9 in, 1 out]
              }
            }
            "Exp 9" <- TRUE
          }
        }
      }
      frame True {
        w837 = 0
      }
    }
    n216 = timed-loop {
      tunnel: w121 -> [w990]
      tunnel: w120 -> [w989]
      tunnel: [w938] -> w119
      tunnel: [w937] -> w118
      timing: w117 -> [_]
      timing-out: [_] -> w116
      tunnel: w115 -> [w924]
      tunnel: w114 -> [w928]
      tunnel: w113 -> [w927]
      tunnel: [w923] -> w112
      tunnel: [w922] -> w111
      tunnel: [w904] -> w110
      tunnel: w101 -> [w919]
      tunnel: w100 -> [w853]
      tunnel: w99 -> [w869]
      tunnel: w109 -> [w908]
      tunnel: w108 -> [w907]
      tunnel: w107 -> [w906]
      tunnel: w106 -> [w905]
      shift-right: [w870] -> _
      shift-left: _ -> [w899]
      tunnel: [w902] -> w105
      tunnel: [w901] -> w104
      tunnel: ["Stop everything"] -> w102
      tunnel: "Automated Experiments or Direct Control" -> [w871]
      tunnel: w93 -> [w864]
      tunnel: w92 -> [w863]
      tunnel: [w862] -> w91
      tunnel: [w861] -> w90
      i -> [w890]
      stop <- w897 stop-if-true
      w841 = 7.5 ("Safety Shut Down Pressure (barg)")
      w920 = 180
      # "in case out of range changes conc to within possible range"
      # "1st 4 flowrates\n5,6 temperatures\n7 pressure (1)\n8 gas (1)"
      # "temperature or syringe or pressure"
      # "We are graphing in barg"
      # "temperature or syringe"
      # "Empty Syringe has level of 50"
      n217 = node-c288() -> ()  [unwired: 1 in, 1 out]
      n218 = call-poly <vilib>:"DAQmx Read.vi"("task/channels in"=w864, "error in"=w863) -> ("task out"=w862:refnum<k21>, "data"=w857:dbl, "error out"=w861:errorcluster)  [unwired: 11 in]
      n219 = Multiply(x=5.1522, y=w857) -> (x*y=w860:dbl)
      n220 = Add(x=-2.6852, y=w860) -> (x+y=w842:dbl)
      "Liquid Inlet Pressure (bar g)" <- w842
      n221 = Greater?(x=w853, y=60) -> (0:w854:bool)
      n222 = Less?(x=w853, y=0) -> (x < y?=w851:bool)
      n223 = case shown="False" w854 {
        tunnel: [w994 1] -> w850
        tunnel: w853 -> [w994 _]
        frame False {
        }
        frame True {
        }
      }
      n224 = case shown="False" w851 {
        tunnel: [w992 1] -> w849
        tunnel: w850 -> [w992 _]
        frame False {
        }
        frame True {
        }
      }
      n225 = for {
        N: 4 -> [_]
        tunnel: w990 -> [w1264] mode=indexing
        tunnel: [w1262] -> w984 mode=indexing
        tunnel: [w1259] -> w979 mode=indexing
        tunnel: [w1258] -> w978 mode=indexing
        tunnel: [w1257] -> w977 mode=indexing
        tunnel: w989 -> [w1256] mode=indexing
        i -> [w1263]
        n226 = call "NCS_GetFlowRateIs.vi"("error in (no error)"=w1256, "dosingunit"=w1263, "device handle in"=w1264) -> ("error out"=w1260:errorcluster, "flowrate is"=w1262:dbl, "device handle out"=w1261:u32)
        n227 = call "NCS_GetSyringeLevelIs.vi"("error in (no error)"=w1260, "dosingunit"=w1263, "device handle in"=w1261) -> ("error out"=w1257:errorcluster, "syringe level is"=w1259:dbl, "device handle out"=w1258:u32)
      }
      n228 = Index Array(array=w979, index=0) -> (element=w894:dbl)
      "Syringe Level 1" <- w894
      n229 = Index Array(array=w979, index=3) -> (element=w891:dbl)
      "Syringe Level 4" <- w891
      n230 = Index Array(array=w979, index=1) -> (element=w893:dbl)
      "Syringe Level 2" <- w893
      n231 = Index Array(array=w979, index=2) -> (element=w892:dbl)
      "Syringe Level 3" <- w892
      n232 = case shown="True" "Shut down in empty?\nLeft off, right on" {
        tunnel: [FALSE w1165] -> w895
        tunnel: w894 -> [_ w1164]
        tunnel: w893 -> [_ w1163]
        tunnel: w892 -> [_ w1162]
        tunnel: w891 -> [_ w1161]
        frame False {
        }
        frame True {
          w1166 = 50
          n233 = Less Or Equal?(x=w1163, y=w1166) -> (x <= y?=w1172:bool)
          n234 = Less Or Equal?(x=w1164, y=w1166) -> (x <= y?=w1167:bool)
          n235 = Less Or Equal?(x=w1162, y=w1166) -> (x <= y?=w1170:bool)
          n236 = Less Or Equal?(x=w1161, y=w1166) -> (x <= y?=w1168:bool)
          n237 = Or(x=w1167, y=w1172) -> (x .or. y?=w1171:bool)
          n238 = Or(x=w1171, y=w1170) -> (x .or. y?=w1169:bool)
          n239 = Or(x=w1169, y=w1168) -> (x .or. y?=w1165:bool)
        }
      }
      n240 = Index Array(array=w984, index=0) -> (element=w881:dbl)
      "Flowrate 1 Low" <- w881
      n241 = Index Array(array=w984, index=3) -> (element=w846:dbl)
      "Flowrate 4 High" <- w846
      n242 = Index Array(array=w984, index=1) -> (element=w880:dbl)
      "Flowrate 2 Low" <- w880
      n243 = Index Array(array=w984, index=2) -> (element=w847:dbl)
      "Flowrate 3 High" <- w847
      n244 = case shown="True" "Clear" {
        tunnel: w899 -> [w1173 _]
        tunnel: [w1173 w1174] -> w898
        frame False {
        }
        frame True {
          n245 = Initialize Array(0, 1) -> (w1174:i32[])
        }
      }
      n246 = call-poly <vilib>:"DAQmx Read.vi"("task/channels in"=w908, "error in"=w907) -> ("task out"=w902:refnum<k21>, "data"=w913:dbl[], "error out"=w901:errorcluster)  [unwired: 11 in]
      n247 = Add(x=w881, y=w880) -> (x+y=w848:dbl)
      n248 = Add(x=w848, y=w847) -> (x+y=w883:dbl)
      n249 = Index Array(array=w913, index=0) -> (element=w911:dbl)
      n250 = Add(x=w883, y=w846) -> (x+y=w882:dbl)
      "Total Flowrate (uL/min)" <- w882
      n251 = Divide(x=w848, y=w882) -> (x/y=w875:dbl)
      n252 = Multiply(x=w911, y=w906) -> (x*y=w912:dbl)
      n253 = Multiply(x="Low Conc", y=w875) -> (x*y=w879:dbl)
      n254 = Add(x=w912, y=w905) -> (x+y=w909:dbl)
      n255 = Add(x=w847, y=w846) -> (x+y=w845:dbl)
      n256 = Divide(x=w845, y=w882) -> (x/y=w876:dbl)
      n257 = Multiply(x="High Conc", y=w876) -> (x*y=w878:dbl)
      n258 = Add(x=w879, y=w878) -> (x+y=→"Feed Concentration (M)":dbl)
      n259 = In Range and Coerce(upper limit="High Conc", x=w869, lower limit="Low Conc") -> (coerced(x)=w866:dbl, In Range?=w868:bool)
      n260 = case shown="False" w868 {
        tunnel: [w997 w999] -> w867
        tunnel: w869 -> [_ w999]
        tunnel: w866 -> [w997 _]
        tunnel: [TRUE FALSE] -> w865
        frame False {
        }
        frame True {
        }
      }
      "Desired Conc Not Possible" <- w865
      n261 = Multiply(x=w909, y=0.0689476) -> (x*y=w856:dbl)
      "Gas Back Pressure (barg)" <- w856
      n262 = case shown="False" w871 {
        tunnel: [w1236 w1237] -> w975
        tunnel: w849 -> [w1230 _]
        tunnel: w867 -> [w1233 _]
        tunnel: "High Conc" -> [w1235 _]
        tunnel: "Low Conc" -> [w1234 _]
        frame False {
          # "h-s/h-l"
          # "s-l/h-l"
          # "high flow"
          # "low flow"
          # "2 syringes each"
          # "h-s"
          # "s-l"
          # "h-l"
          n263 = Subtract(x=w1235, y=w1234) -> (x-y=w1223:dbl)
          n264 = Subtract(x=w1233, y=w1234) -> (x-y=w1232:dbl)
          n265 = Subtract(x=w1235, y=w1233) -> (x-y=w1224:dbl)
          n266 = Divide(x=w1230, y=2) -> (x/y=w1229:dbl)
          n267 = Divide(x=w1224, y=w1223) -> (x/y=w1228:dbl)
          n268 = Divide(x=w1232, y=w1223) -> (x/y=w1227:dbl)
          n269 = Multiply(x=w1229, y=w1228) -> (x*y=w1226:dbl)
          n270 = Multiply(x=w1229, y=w1227) -> (x*y=w1225:dbl)
          n271 = Build Array(w1226, w1226, w1225, w1225) -> (w1236:dbl[])
        }
        frame True {
          n272 = Build Array("Set Flowrate 1", "Set Flowrate 2", "Set Flowrate 3", "Set Flowrate 4") -> (w1237:dbl[])
        }
      }
      n273 = Greater Or Equal?(x=w842, y=w841) -> (x >= y?=w840:bool)
      n274 = Build Array (concatenate)(w898, w856) -> (w870:dbl[])
      "Calculated Pressure" <- w870
      n275 = Greater Or Equal?(x=w856, y=w841) -> (x >= y?=w839:bool)
      n276 = Or(x=w840, y=w839) -> (x .or. y?=w838:bool)
      n277 = case shown="True" w871 {
        tunnel: [w1178 FALSE] -> w873
        tunnel: w890 -> [w1177 _]
        frame False {
          # "changes set points for each new exp"
          n278 = Equal?(x=w1177, y=0) -> (x = y?=w1178:bool)
        }
        frame True {
          # "at end of each exp"
          # "doesnt automatically change set point"
        }
      }
      n279 = Or(x=w873, y="Update Temperature Set Point") -> (x .or. y?=w930:bool)
      n280 = case shown="True" w930 {
        tunnel: w928 -> [w1182 w1190]
        tunnel: w927 -> [w1181 w1189]
        tunnel: [w1182 w1188] -> w926
        tunnel: [w1181 w1187] -> w925
        tunnel: w924 -> [_ w1186]
        tunnel: w871 -> [_ w1184]
        tunnel: w919 -> [_ w1183]
        frame False {
        }
        frame True {
          n281 = case shown="False" w1184 {
            tunnel: [w1191 "Set Point (oC)"] -> w1185
            tunnel: w1183 -> [w1191 _]
            frame False {
            }
            frame True {
            }
          }
          n282 = call "CN7500_Write Set Point Value.vi"("Target Set Point Value"=w1185, "error in (no error)"=w1189, "Controller Number"=w1186, "VISA In"=w1190) -> ("error out"=w1187:errorcluster, "VISA Out"=w1188:refnum<visa-resource-name>)  [unwired: 6 in]
        }
      }
      n283 = Or(x="Generate Flow", y=w873) -> (x .or. y?=w874:bool)
      n284 = case shown="True" w874 {
        tunnel: w978 -> [w1243 w1248]
        tunnel: w977 -> [w1242 w1247]
        tunnel: [w1242 w1246] -> w885
        tunnel: [w1243 w1245] -> w884
        tunnel: w975 -> [_ w1244]
        frame False {
        }
        frame True {
          n285 = for {
            N: 4 -> [_]
            tunnel: w1248 -> [w1255] mode=indexing
            tunnel: w1247 -> [w1254] mode=indexing
            tunnel: [w1253] -> w1246 mode=indexing
            tunnel: [w1252] -> w1245 mode=indexing
            tunnel: w1244 -> [w1250] mode=indexing
            i -> [w1251]
            n286 = call "NCS_GenerateFlow.vi"("error in (no error)"=w1254, "flowrate"=w1250, "dosingunit"=w1251, "device handle in"=w1255) -> ("error out"=w1253:errorcluster, "device handle out"=w1252:u32)
          }
        }
      }
      n287 = call "CN7500_Read Process Value.vi"("error in (no error)"=w925, "Controller Number"=w924, "VISA In"=w926) -> ("error out"=w923:errorcluster, "Set Point Value"=w915:dbl, "Process Value"=w916:dbl, "VISA Out"=w922:refnum<visa-resource-name>)  [unwired: 5 in]
      "Temp Set Point (oC)" <- w915
      "Actual Temp (oC)" <- w916
      n288 = Merge Signals(w916, w915) -> (→"Temperature":dynamicdata)
      n289 = Merge Signals(w881, w880, w847, w846, w916, w915, w856, w842) -> (w936:dynamicdata)
      n290 = Greater Or Equal?(x=w916, y=w920) -> (x >= y?=w918:bool)
      n291 = call "Write To Measurement File"("Signals"=w936) -> ()  [unwired: 16 in, 3 out]
      n292 = Index Array(array=w885, index=0) -> (element=w965:errorcluster)
      n293 = Index Array(array=w884, index=0) -> (element=w966:u32)
      n294 = Index Array(array=w885, index=3) -> (element=w955:errorcluster)
      n295 = Index Array(array=w885, index=2) -> (element=w957:errorcluster)
      n296 = Index Array(array=w885, index=1) -> (element=w959:errorcluster)
      n297 = Index Array(array=w884, index=3) -> (element=w956:u32)
      n298 = Index Array(array=w884, index=2) -> (element=w958:u32)
      n299 = Index Array(array=w884, index=1) -> (element=w960:u32)
      n300 = case shown="False" "Stop Dose 2" {
        tunnel: w960 -> [w1210 w1215]
        tunnel: w959 -> [w1209 w1214]
        tunnel: [w1210 w1213] -> w952
        tunnel: [w1209 w1212] -> w951
        frame False {
        }
        frame True {
          n301 = call "NCS_Stop.vi"("error in (no error)"=w1214, "dosingunit"=1, "device handle in"=w1215) -> ("error out"=w1212:errorcluster, "device handle out"=w1213:u32)
        }
      }
      n302 = case shown="False" "Stop Dose 1" {
        tunnel: w966 -> [w1217 w1222]
        tunnel: w965 -> [w1216 w1221]
        tunnel: [w1217 w1220] -> w954
        tunnel: [w1216 w1219] -> w953
        frame False {
        }
        frame True {
          n303 = call "NCS_Stop.vi"("error in (no error)"=w1221, "dosingunit"=0, "device handle in"=w1222) -> ("error out"=w1219:errorcluster, "device handle out"=w1220:u32)
        }
      }
      n304 = case shown="False" "Stop Dose 3" {
        tunnel: w958 -> [w1203 w1208]
        tunnel: w957 -> [w1202 w1207]
        tunnel: [w1203 w1206] -> w950
        tunnel: [w1202 w1205] -> w949
        frame False {
        }
        frame True {
          n305 = call "NCS_Stop.vi"("error in (no error)"=w1207, "dosingunit"=2, "device handle in"=w1208) -> ("error out"=w1205:errorcluster, "device handle out"=w1206:u32)
        }
      }
      n306 = case shown="False" "Stop Dose 4" {
        tunnel: w956 -> [w1196 w1201]
        tunnel: w955 -> [w1195 w1200]
        tunnel: [w1196 w1199] -> w948
        tunnel: [w1195 w1198] -> w947
        frame False {
        }
        frame True {
          n307 = call "NCS_Stop.vi"("error in (no error)"=w1200, "dosingunit"=3, "device handle in"=w1201) -> ("error out"=w1198:errorcluster, "device handle out"=w1199:u32)
        }
      }
      n308 = case shown="False" "Safety or Emergency Syringe Control" {
        tunnel: w954 -> [w1007 w1048]
        tunnel: w953 -> [w1003 w1047]
        tunnel: w952 -> [w1006 w1046]
        tunnel: w951 -> [w1002 w1045]
        tunnel: w950 -> [w1005 w1044]
        tunnel: w949 -> [w1001 w1043]
        tunnel: w948 -> [w1004 w1042]
        tunnel: w947 -> [w1000 w1041]
        tunnel: [w1007 w1018] -> w946
        tunnel: [w1006 w1017] -> w945
        tunnel: [w1005 w1016] -> w944
        tunnel: [w1004 w1015] -> w943
        tunnel: [w1002 w1014] -> w942
        tunnel: [w1001 w1013] -> w941
        tunnel: [w1000 w1012] -> w940
        tunnel: [w1003 w1008] -> w939
        frame False {
        }
        frame True {
          n309 = case shown="False" "Calibrate 2" {
            tunnel: w1046 -> [w1147 w1152]
            tunnel: w1045 -> [w1146 w1151]
            tunnel: [w1147 w1150] -> w1035
            tunnel: [w1146 w1149] -> w1034
            frame False {
            }
            frame True {
              n310 = call "NCS_Calibrate.vi"("error in (no error)"=w1151, "dosingunit"=1, "device handle in"=w1152) -> ("error out"=w1149:errorcluster, "device handle out"=w1150:u32)
            }
          }
          n311 = case shown="False" "Calibrate 3" {
            tunnel: w1044 -> [w1140 w1145]
            tunnel: w1043 -> [w1139 w1144]
            tunnel: [w1140 w1143] -> w1033
            tunnel: [w1139 w1142] -> w1032
            frame False {
            }
            frame True {
              n312 = call "NCS_Calibrate.vi"("error in (no error)"=w1144, "dosingunit"=2, "device handle in"=w1145) -> ("error out"=w1142:errorcluster, "device handle out"=w1143:u32)
            }
          }
          n313 = case shown="False" "Calibrate 1" {
            tunnel: w1048 -> [w1154 w1159]
            tunnel: w1047 -> [w1153 w1158]
            tunnel: [w1154 w1157] -> w1037
            tunnel: [w1153 w1156] -> w1036
            frame False {
            }
            frame True {
              n314 = call "NCS_Calibrate.vi"("error in (no error)"=w1158, "dosingunit"=0, "device handle in"=w1159) -> ("error out"=w1156:errorcluster, "device handle out"=w1157:u32)
            }
          }
          n315 = case shown="False" "Calibrate 4" {
            tunnel: w1042 -> [w1133 w1138]
            tunnel: w1041 -> [w1132 w1137]
            tunnel: [w1133 w1136] -> w1031
            tunnel: [w1132 w1135] -> w1030
            frame False {
            }
            frame True {
              n316 = call "NCS_Calibrate.vi"("error in (no error)"=w1137, "dosingunit"=3, "device handle in"=w1138) -> ("error out"=w1135:errorcluster, "device handle out"=w1136:u32)
            }
          }
          n317 = case shown="False" "Empty 2" {
            tunnel: w1035 -> [w1113 w1117]
            tunnel: w1034 -> [w1112 w1115]
            tunnel: [w1113 w1116] -> w1021
            tunnel: [w1112 w1114] -> w1022
            frame False {
            }
            frame True {
              w1119 = 1
              n318 = call "NCS_GetFlowRateMax.vi"("error in (no error)"=w1115, "dosingunit"=w1119, "device handle in"=w1117) -> ("error out"=w1120:errorcluster, "flow rate max"=w1118:dbl, "device handle out"=w1121:u32)
              n319 = call "NCS_EmptySyrige.vi"("error in (no error)"=w1120, "flowrate"=w1118, "dosingunit"=w1119, "device handle in"=w1121) -> ("error out"=w1114:errorcluster, "device handle out"=w1116:u32)
            }
          }
          n320 = case shown="False" "Empty 1" {
            tunnel: w1037 -> [w1123 w1131]
            tunnel: w1036 -> [w1122 w1128]
            tunnel: [w1123 w1129] -> w1019
            tunnel: [w1122 w1126] -> w1020
            frame False {
            }
            frame True {
              w1125 = 0
              n321 = call "NCS_GetFlowRateMax.vi"("error in (no error)"=w1128, "dosingunit"=w1125, "device handle in"=w1131) -> ("error out"=w1127:errorcluster, "flow rate max"=w1124:dbl, "device handle out"=w1130:u32)
              n322 = call "NCS_EmptySyrige.vi"("error in (no error)"=w1127, "flowrate"=w1124, "dosingunit"=w1125, "device handle in"=w1130) -> ("error out"=w1126:errorcluster, "device handle out"=w1129:u32)
            }
          }
          n323 = case shown="False" "Empty 3" {
            tunnel: w1033 -> [w1103 w1104]
            tunnel: w1032 -> [w1102 w1105]
            tunnel: [w1103 w1106] -> w1023
            tunnel: [w1102 w1107] -> w1024
            frame False {
            }
            frame True {
              w1109 = 2
              n324 = call "NCS_GetFlowRateMax.vi"("error in (no error)"=w1105, "dosingunit"=w1109, "device handle in"=w1104) -> ("error out"=w1110:errorcluster, "flow rate max"=w1108:dbl, "device handle out"=w1111:u32)
              n325 = call "NCS_EmptySyrige.vi"("error in (no error)"=w1110, "flowrate"=w1108, "dosingunit"=w1109, "device handle in"=w1111) -> ("error out"=w1107:errorcluster, "device handle out"=w1106:u32)
            }
          }
          n326 = case shown="False" "Empty 4" {
            tunnel: w1031 -> [w1093 w1094]
            tunnel: w1030 -> [w1092 w1095]
            tunnel: [w1093 w1097] -> w1025
            tunnel: [w1092 w1096] -> w1026
            frame False {
            }
            frame True {
              w1099 = 3
              n327 = call "NCS_GetFlowRateMax.vi"("error in (no error)"=w1095, "dosingunit"=w1099, "device handle in"=w1094) -> ("error out"=w1100:errorcluster, "flow rate max"=w1098:dbl, "device handle out"=w1101:u32)
              n328 = call "NCS_EmptySyrige.vi"("error in (no error)"=w1100, "flowrate"=w1098, "dosingunit"=w1099, "device handle in"=w1101) -> ("error out"=w1096:errorcluster, "device handle out"=w1097:u32)
            }
          }
          n329 = case shown="False" "Refill 2" {
            tunnel: w1021 -> [w1073 w1077]
            tunnel: w1022 -> [w1072 w1075]
            tunnel: [w1073 w1076] -> w1017
            tunnel: [w1072 w1074] -> w1014
            frame False {
            }
            frame True {
              w1079 = 1
              n330 = call "NCS_GetFlowRateMax.vi"("error in (no error)"=w1075, "dosingunit"=w1079, "device handle in"=w1077) -> ("error out"=w1080:errorcluster, "flow rate max"=w1078:dbl, "device handle out"=w1081:u32)
              n331 = call "NCS_RefillSyrige.vi"("error in (no error)"=w1080, "flowrate"=w1078, "dosingunit"=w1079, "device handle in"=w1081) -> ("error out"=w1074:errorcluster, "device handle out"=w1076:u32)
            }
          }
          n332 = case shown="False" "Refill 1" {
            tunnel: w1019 -> [w1083 w1091]
            tunnel: w1020 -> [w1082 w1088]
            tunnel: [w1083 w1089] -> w1018
            tunnel: [w1082 w1086] -> w1008
            frame False {
            }
            frame True {
              w1085 = 0
              n333 = call "NCS_GetFlowRateMax.vi"("error in (no error)"=w1088, "dosingunit"=w1085, "device handle in"=w1091) -> ("error out"=w1087:errorcluster, "flow rate max"=w1084:dbl, "device handle out"=w1090:u32)
              n334 = call "NCS_RefillSyrige.vi"("error in (no error)"=w1087, "flowrate"=w1084, "dosingunit"=w1085, "device handle in"=w1090) -> ("error out"=w1086:errorcluster, "device handle out"=w1089:u32)
            }
          }
          n335 = case shown="False" "Refill 3" {
            tunnel: w1023 -> [w1063 w1064]
            tunnel: w1024 -> [w1062 w1065]
            tunnel: [w1063 w1066] -> w1016
            tunnel: [w1062 w1067] -> w1013
            frame False {
            }
            frame True {
              w1069 = 2
              n336 = call "NCS_GetFlowRateMax.vi"("error in (no error)"=w1065, "dosingunit"=w1069, "device handle in"=w1064) -> ("error out"=w1070:errorcluster, "flow rate max"=w1068:dbl, "device handle out"=w1071:u32)
              n337 = call "NCS_RefillSyrige.vi"("error in (no error)"=w1070, "flowrate"=w1068, "dosingunit"=w1069, "device handle in"=w1071) -> ("error out"=w1067:errorcluster, "device handle out"=w1066:u32)
            }
          }
          n338 = case shown="False" "Refill 4" {
            tunnel: w1025 -> [w1053 w1054]
            tunnel: w1026 -> [w1052 w1055]
            tunnel: [w1053 w1057] -> w1015
            tunnel: [w1052 w1056] -> w1012
            frame False {
            }
            frame True {
              w1059 = 3
              n339 = call "NCS_GetFlowRateMax.vi"("error in (no error)"=w1055, "dosingunit"=w1059, "device handle in"=w1054) -> ("error out"=w1060:errorcluster, "flow rate max"=w1058:dbl, "device handle out"=w1061:u32)
              n340 = call "NCS_RefillSyrige.vi"("error in (no error)"=w1060, "flowrate"=w1058, "dosingunit"=w1059, "device handle in"=w1061) -> ("error out"=w1056:errorcluster, "device handle out"=w1057:u32)
            }
          }
        }
      }
      n341 = Or(x=w918, y=w895) -> (x .or. y?=w903:bool)
      n342 = Or(x=w903, y=w838) -> (x .or. y?=w904:bool)
      n343 = Multiply(x="Minutes between Exp", y=60) -> (x*y=w887:dbl)
      n344 = Divide(x=w887, y=5) -> (x/y=w888:dbl)
      n345 = Greater Or Equal?(x=w890, y=w888) -> (x >= y?=w932:bool)
      n346 = Or(x=w932, y=w904) -> (x .or. y?=w917:bool)
      n347 = Or(x="Skip Exp", y=w917) -> (x .or. y?=w933:bool)
      n348 = Or(x="Stop everything", y=w933) -> (x .or. y?=w897:bool)
      n349 = node-c288() -> ()  [unwired: 1 in, 1 out]
      n350 = Build Array(w946, w945, w944, w943) -> (w938:u32[])
      n351 = Build Array(w939, w942, w941, w940) -> (w937:errorcluster[])
      "loop ind" <- w890
      "Safety Shut Down Temp" <- w920
      "Safety Shut Down Pressure (barg)" <- w841
    }
    n352 = Or(x=w102, y=w110) -> (x .or. y?=w103:bool)
    n353 = node-c288(w116) -> ()  [unwired: 1 out]
    "HPLC file name, MBDoE2peakin1" <- w87
    "Record filename, RecordAmbInitisileFactorial1MD" <- w86
  }
  n354 = call <vilib>:"DAQmx Stop Task.vi"("task/channels in"=w19, "error in"=w18) -> ("task out"=w21:refnum<k21>, "error out"=w20:errorcluster)  [unwired: 12 in]
  n355 = Index Array(array=w48, index=0) -> (element=w50:u32)
  n356 = Index Array(array=w47, index=0) -> (element=w49:errorcluster)
  n357 = call <vilib>:"DAQmx Stop Task.vi"("task/channels in"=w8, "error in"=w6) -> ("task out"=w7:refnum<k21>, "error out"=w9:errorcluster)  [unwired: 12 in]
  n358 = call <vilib>:"DAQmx Clear Task.vi"("task in"=w21, "error in"=w20) -> ()  [unwired: 13 in, 1 out]
  n359 = call <vilib>:"DAQmx Clear Task.vi"("task in"=w7, "error in"=w9) -> ()  [unwired: 13 in, 1 out]
  n360 = call "NCS_CloseDevice.vi"("error in (no error)"=w49, "device handle"=w50) -> ()  [unwired: 1 out]
  n361 = call "CN7500_Write Set Point Value.vi"("Target Set Point Value"=25, "error in (no error)"=w36, "Controller Number"=w39, "VISA In"=w35) -> ("error out"=w41:errorcluster, "VISA Out"=w42:refnum<visa-resource-name>)  [unwired: 6 in]
  n362 = call "CN7500_Close.vi"("error in (no error)"=w41, "VISA resource name"=w42) -> ()  [unwired: 9 in, 1 out]
